vi "Main - bkp.vi"() -> ()   [LabVIEW 2013]
uses:
  <vilib>/Utility/error.llb/DialogType.ctl
  <vilib>/Utility/miscctls.llb/LVFontTypeDef.ctl
panel:
  out "Buv con ID":refnum<k5>
  out "LoadVolt":bool
  out "LoadPhase":bool
  in  "Tab Control":enum32{"ЛИНЗЫ ПОСТ. ТОКА", "ЛИНЗЫ ИМПУЛЬСНЫЕ"}(tab)
  in  "List of channels":i32(listbox)
  in  "ReadFromFile":bool
  in  "WriteToFile":bool
  out "Дата":string
  out "Время":string
  in  "Comm. current %":dbl=0.5 caption="А" min=0.0 max=72.0 step=0.25
  in  "Common curr. dec":bool
  in  "Common curr. inc":bool
  in  "ConnectAll":bool
  in  "DisconnectAll":bool
  in  "Set Output ON All":bool caption="ВЫХОДЫ ИСТОЧНИКОВ"
  out "текущий ист.":u8
  in  "SetCurrent":dbl min=0.0 max=72.0 step=0.1 format="%#.1g"
  in  "SetVoltage":dbl min=0.0 max=30.0 step=0.1 format="%#.1g"
  in  "SetCurrentB":bool
  in  "SetVoltageB":bool
  in  "SetOutputOffB":bool
  in  "SetOutputOnB":bool
  in  "ConnectChannel":bool
  in  "DisconnectChannel":bool
  in  "SetPhaseEn":bool=TRUE
  in  "BuvPhaseSetB":bool
  in  "SelectedBuvPhase":u16=7000 max=1000 step=1
  out "текущий ист. БУВ":u8
  in  "SelectedBuvOutVolt":dbl min=0.0 max=1000.0 step=0.1 format="%.1f"
  in  "SelectedBuvSetVolB":bool
  in  "Buv Table":i32(listbox)
  in  "Quit":bool=TRUE
  in  "SetCurrentAll":bool
  in  "SetVoltageAll":bool
  in  "Comm. voltage %":dbl caption="%" min=0.0 max=100.0 step=0.5
  in  "Common volt. dec":bool
  in  "Common volt. inc":bool
  in  "№":string="55"
  in  "DeleteChannel":bool
  in  "IP":string="172.16.21.19"
  in  "AddChannel":bool
  out "CURRENTSET":dbl[](array[numeric])
  in  "CurrentModulationOn":bool
  in  "Amp":dbl
  in  "CurrentModulationB":bool
  out "NAME":string[](array[string])
  out "ADRESS":string[](array[string])
  out "Measure_VI":refnum<vi>[](array[refnum])
  # "ВСЕ ИСТОЧНИКИ"
  # "ИСТОЧНИК №_"
  # "ИСТОЧНИК №_"
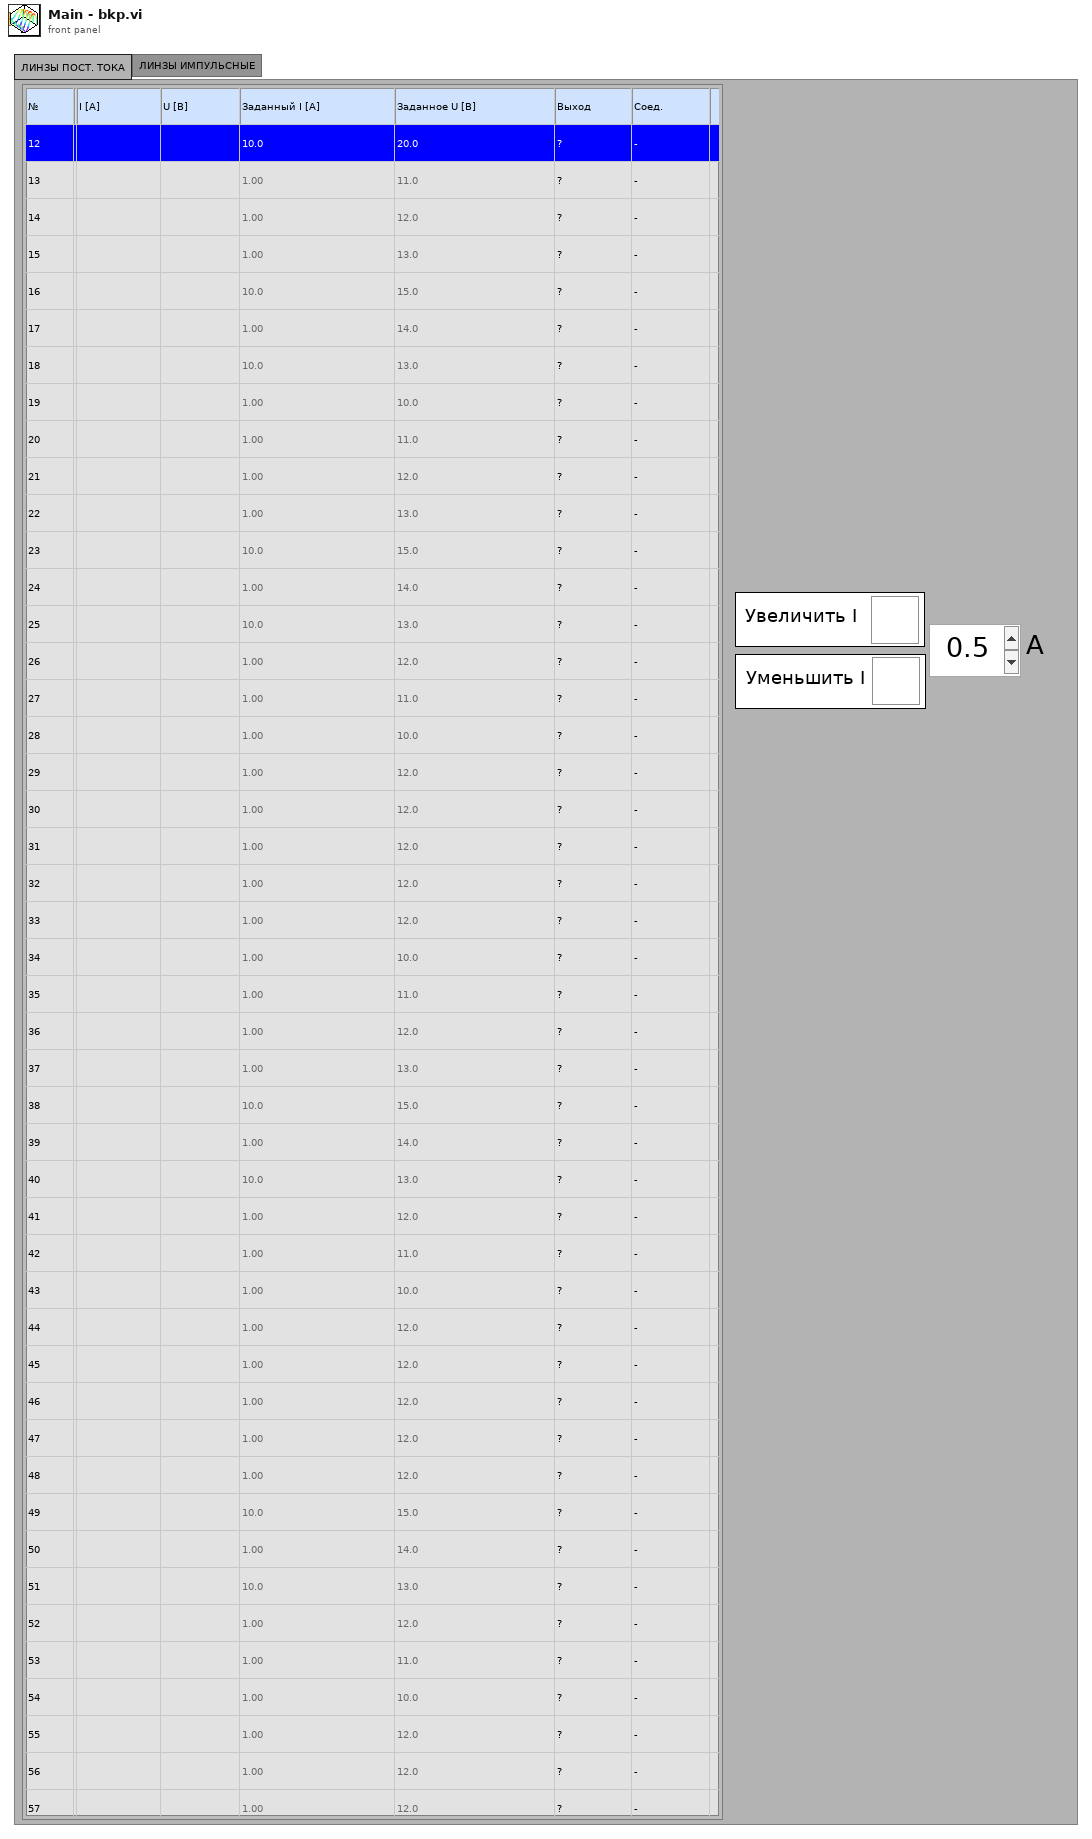
[diagram p1: front panel]
types:
  T1 = enum16{"open", "replace", "create", "open or create", "replace or create", "replace or create with confirmation"}
  T2 = enum8{"Enabled", "Disabled", "Disabled and Grayed Out"}
  T3 = typedef "DialogType.ctl" = u16
  T4 = typedef "LVFontTypeDef.ctl" = cluster{"Font Name":string, "Size":u16, "Bold":bool, "Italic":bool, "Underline":bool, "Strikeout":bool, "Color":u32}
  T5 = enum16{"Standard", "Buffered", "CRLF", "Immediate"}
  T6 = cluster{"milliseconds to wait":i32, "milliseconds to wait":i32}
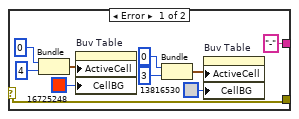
[diagram p6: hidden frame]
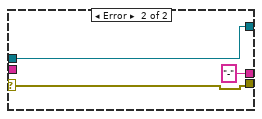
[diagram p7: hidden frame]
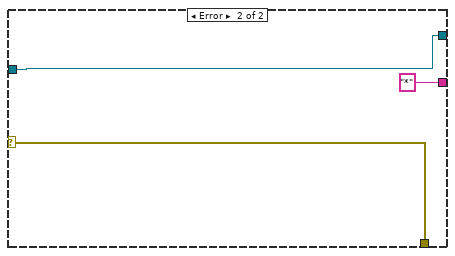
[diagram p8: hidden frame]
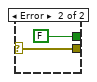
[diagram p10: hidden frame]
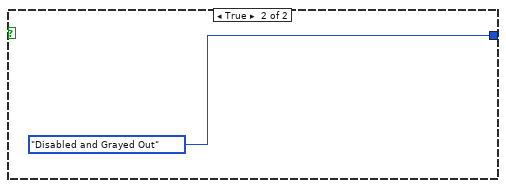
[diagram p11: hidden frame]
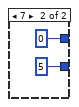
[diagram p13: hidden frame]
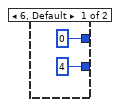
[diagram p14: hidden frame]
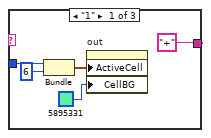
[diagram p15: hidden frame]
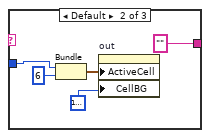
[diagram p16: hidden frame]
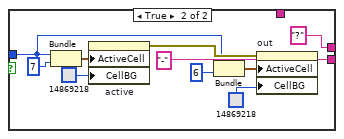
[diagram p17: hidden frame]
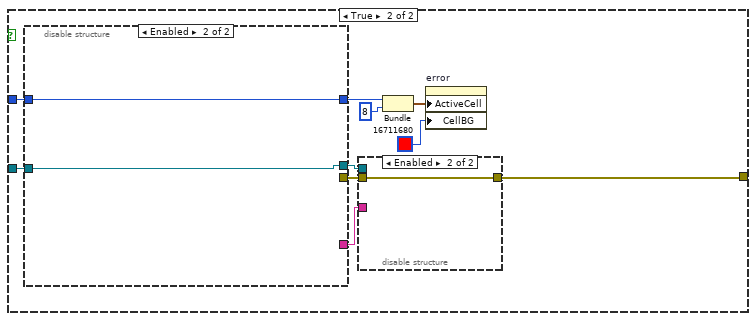
[diagram p18: hidden frame]
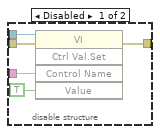
[diagram p19: hidden frame]
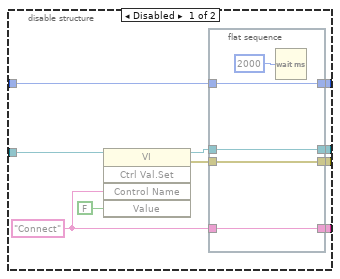
[diagram p20: hidden frame]
diagram:
  w38 = u8 0 ("Disabled")
  w40 = FALSE ("SetOutputOnB")
  w41 = FALSE ("OK Button")
  n1 = event shown="[0] \"Quit\": Value Change" {
    selector: _ -> [_]
    dyn-events: _ -> [_]
    timeout: _ -> [_]
    event "Quit": Value Change {
      n2 = event-data() -> ()  [unwired: 1 in, 1 out]
      n3 = flat-sequence {
        frame #0 {
          w46 = T3 0 items=["no dialog", "OK message", "continue or stop message", "OK message + warnings", "continue/stop + warnings"] ("type of dialog (OK msg:1)")
          n4 = local read "Measure_VI"() -> (w52:refnum<vi>[])
          n5 = local read "Buv con ID"() -> (w50:refnum<k5>)
          n6 = Array Size(array=w52) -> (size(s)=w51:i32)
          n7 = for {
            N: w51 -> [_]
            tunnel: [w53] -> w49 mode=indexing
            i -> [w54]
            n8 = local read "Measure_VI"() -> (w57:refnum<vi>[])
            n9 = Index Array(array=w57, index=w54) -> (element=w56:refnum<vi>)
            n10 = invoke class="VI" method="Ctrl Val.Set"(reference=w56, "Control Name"="Connect", "Value"=FALSE ("OK Button")) -> (error out=w53:errorcluster)  [unwired: 2 in, 4 out]
          }
          n11 = TCP Close Connection(connection ID=w50) -> (error out=w48:errorcluster)  [unwired: 2 in, 1 out]
          n12 = Merge Errors(w49, w48) -> (w47:errorcluster)
          n13 = call <vilib>:"General Error Handler.vi"("type of dialog (OK msg:1)"=w46, "error in (no error)"=w47) -> ()  [unwired: 9 in, 5 out]
        }
        frame #1 {
        }
        frame #2 {
          n14 = Stop(stop? (T)=TRUE) -> ()
        }
      }
    }
  }
  n15 = while {
    stop <- FALSE stop-if-true
    n16 = property on="List of channels" class="MCListbox (strict)"() -> ("ItemNames"=w66:string[][])  [unwired: 2 in, 2 out]
    n17 = Get Date/Time String(want seconds? (F)=TRUE) -> (date string=→"Дата":string, time string=→"Время":string)  [unwired: 2 in]
    n18 = Wait Until Next ms Multiple(millisecond multiple=u16 1000) -> ()  [unwired: 1 out]
    n19 = Empty Array?(array=w66) -> (empty?=w65:bool)
    n20 = case shown="False" w65 {
      tunnel: [T2."Enabled" ("Disabled") T2."Disabled and Grayed Out" ("Disabled")] -> w60
      frame False {
      }
      frame True {
      }
    }
    n21 = property on="Common curr. inc" class="Bool (strict)"("DisabledEnum"=w60) -> ()  [unwired: 2 in, 2 out]
    n22 = property on="Common curr. dec" class="Bool (strict)"("DisabledEnum"=w60) -> ()  [unwired: 2 in, 2 out]
    n23 = property on="Set Output ON All" class="Bool (strict)"("DisabledEnum"=w60) -> ()  [unwired: 2 in, 2 out]
    n24 = property on="Common volt. inc" class="Bool (strict)"("DisabledEnum"=w60) -> ()  [unwired: 2 in, 2 out]
    n25 = property on="DisconnectAll" class="Bool (strict)"("DisabledEnum"=w60) -> ()  [unwired: 2 in, 2 out]
    n26 = property on="SetVoltageB" class="Bool (strict)"("DisabledEnum"=w60) -> ()  [unwired: 2 in, 2 out]
    n27 = property on="ConnectChannel" class="Bool (strict)"("DisabledEnum"=w60) -> ()  [unwired: 2 in, 2 out]
    n28 = property on="SetOutputOnB" class="Bool (strict)"("DisabledEnum"=w60) -> ()  [unwired: 2 in, 2 out]
    n29 = property on="DisconnectChannel" class="Bool (strict)"("DisabledEnum"=w60) -> ()  [unwired: 2 in, 2 out]
    n30 = property on="SetOutputOffB" class="Bool (strict)"("DisabledEnum"=w60) -> ()  [unwired: 2 in, 2 out]
    n31 = property on="ConnectAll" class="Bool (strict)"("DisabledEnum"=w60) -> ()  [unwired: 2 in, 2 out]
    n32 = property on="SetCurrentB" class="Bool (strict)"("DisabledEnum"=w60) -> ()  [unwired: 2 in, 2 out]
  }
  n33 = while {
    stop <- FALSE stop-if-true
    n34 = event shown="[16] \"WriteToFile\": Value Change" {
      selector: _ -> [_ _ _ _ _ _ _ _ _ _ _ _ _ _ _ _ _ _ _ _]
      dyn-events: _ -> [_ _ _ _ _ _ _ _ _ _ _ _ _ _ _ _ _ _ _ _]
      timeout: _ -> [_ _ _ _ _ _ _ _ _ _ _ _ _ _ _ _ _ _ _ _]
      tunnel: [w73 _ _ _ w177 w193 w209 w250 w291 w306 w332 w348 w364 w381 w402 w425 w443 w494 w571 w594] -> w70
      event "AddChannel": Value Change {
        n35 = event-data() -> ()  [unwired: 7 out]
        n36 = flat-sequence {
          tunnel: [w76] -> w74
          tunnel: [w86] -> w73
          tunnel: w74 -> [w86]
          frame #0 {
            w75 = u8 2 ("Disabled")
            n37 = property on="Quit" class="Bool (strict)"("Disabled"=w75) -> ()  [unwired: 2 in, 2 out]
            n38 = property on="AddChannel" class="Bool (strict)"("Disabled"=w75) -> ()  [unwired: 2 in, 2 out]
            n39 = property on="CurrentModulationB" class="Bool (strict)"("Disabled"=w75) -> ()  [unwired: 2 in, 2 out]
            n40 = property on="DisconnectChannel" class="Bool (strict)"("Disabled"=w75) -> ()  [unwired: 2 in, 2 out]
            n41 = property on="ConnectAll" class="Bool (strict)"("Disabled"=w75) -> ()  [unwired: 2 in, 2 out]
            n42 = property on="ReadFromFile" class="Bool (strict)"("Disabled"=w75) -> ()  [unwired: 2 in, 2 out]
            n43 = property on="ConnectChannel" class="Bool (strict)"("Disabled"=w75) -> ()  [unwired: 2 in, 2 out]
            n44 = property on="DeleteChannel" class="Bool (strict)"("Disabled"=w75) -> ()  [unwired: 2 in, 2 out]
            n45 = property on="SetOutputOnB" class="Bool (strict)"("Disabled"=w75) -> ()  [unwired: 2 in, 2 out]
            n46 = property on="Set Output ON All" class="Bool (strict)"("Disabled"=w75) -> ()  [unwired: 2 in, 2 out]
            n47 = property on="SetVoltageB" class="Bool (strict)"("Disabled"=w75) -> ()  [unwired: 2 in, 2 out]
            n48 = property on="SetOutputOffB" class="Bool (strict)"("Disabled"=w75) -> ()  [unwired: 2 in, 2 out]
            n49 = property on="SetVoltageAll" class="Bool (strict)"("Disabled"=w75) -> ()  [unwired: 2 in, 2 out]
            n50 = property on="SetCurrentAll" class="Bool (strict)"("Disabled"=w75) -> ()  [unwired: 2 in, 2 out]
            n51 = property on="DisconnectAll" class="Bool (strict)"("Disabled"=w75) -> ()  [unwired: 2 in, 2 out]
            n52 = property on="WriteToFile" class="Bool (strict)"("Disabled"=w75) -> ()  [unwired: 2 in, 2 out]
            n53 = property on="SetCurrentB" class="Bool (strict)"("Disabled"=w75) -> ()  [unwired: 2 in, 2 out]
          }
          frame #1 {
            w77 = 0.0 ("SetVoltage")
            n54 = local read "Measure_VI"() -> (w81:refnum<vi>[])
            n55 = local read "ADRESS"() -> (w83:string[])
            n56 = local read "NAME"() -> (w82:string[])
            n57 = call "AddChannel.vi"("VIRef"=w81, "Name"="№", "SetCurrent"=w77, "ADRESS"=w83, "NAME"=w82, "Address"="IP", "SetVoltage"=w77) -> ("NAMEOut"=w78:string[], "error out"=w76:errorcluster, "ADRESSOut"=w79:string[], "VIRefOut"=w80:refnum<vi>[])  [unwired: 1 in, 4 out]
            n58 = local write "NAME"(w78) -> ()
            n59 = local write "ADRESS"(w79) -> ()
            n60 = local write "Measure_VI"(w80) -> ()
          }
          frame #2 {
            w87 = u8 0 ("Disabled")
            n61 = local write "AddChannel"(FALSE ("AddChannel")) -> ()
            n62 = property on="Quit" class="Bool (strict)"("Disabled"=w87) -> ()  [unwired: 2 in, 2 out]
            n63 = property on="AddChannel" class="Bool (strict)"("Disabled"=w87) -> ()  [unwired: 2 in, 2 out]
            n64 = property on="CurrentModulationB" class="Bool (strict)"("Disabled"=w87) -> ()  [unwired: 2 in, 2 out]
            n65 = property on="DisconnectChannel" class="Bool (strict)"("Disabled"=w87) -> ()  [unwired: 2 in, 2 out]
            n66 = property on="ReadFromFile" class="Bool (strict)"("Disabled"=w87) -> ()  [unwired: 2 in, 2 out]
            n67 = property on="ConnectChannel" class="Bool (strict)"("Disabled"=w87) -> ()  [unwired: 2 in, 2 out]
            n68 = property on="DeleteChannel" class="Bool (strict)"("Disabled"=w87) -> ()  [unwired: 2 in, 2 out]
            n69 = property on="SetVoltageB" class="Bool (strict)"("Disabled"=w87) -> ()  [unwired: 2 in, 2 out]
            n70 = property on="Set Output ON All" class="Bool (strict)"("Disabled"=w87) -> ()  [unwired: 2 in, 2 out]
            n71 = property on="SetOutputOffB" class="Bool (strict)"("Disabled"=w87) -> ()  [unwired: 2 in, 2 out]
            n72 = property on="ConnectAll" class="Bool (strict)"("Disabled"=w87) -> ()  [unwired: 2 in, 2 out]
            n73 = property on="SetVoltageAll" class="Bool (strict)"("Disabled"=w87) -> ()  [unwired: 2 in, 2 out]
            n74 = property on="SetCurrentAll" class="Bool (strict)"("Disabled"=w87) -> ()  [unwired: 2 in, 2 out]
            n75 = property on="DisconnectAll" class="Bool (strict)"("Disabled"=w87) -> ()  [unwired: 2 in, 2 out]
            n76 = property on="WriteToFile" class="Bool (strict)"("Disabled"=w87) -> ()  [unwired: 2 in, 2 out]
            n77 = property on="SetCurrentB" class="Bool (strict)"("Disabled"=w87) -> ()  [unwired: 2 in, 2 out]
            n78 = property on="SetOutputOnB" class="Bool (strict)"("Disabled"=w87) -> ()  [unwired: 2 in, 2 out]
          }
        }
      }
      event "List of channels": Mouse Down {
        # "Работа с выбранным источником"
        n79 = event-data() -> ()  [unwired: 2 out]
        n80 = property on="List of channels" class="MCListbox (strict)"() -> ("ItemNames"=w92:string[][])  [unwired: 2 in, 2 out]
        n81 = property on="List of channels" class="MCListbox (strict)"() -> ("Value"=w91:i32)  [unwired: 2 in, 2 out]
        n82 = Index Array(array=w92, index (row)=w91) -> (element=w90:string[])  [unwired: 1 in]
        n83 = Empty Array?(array=w90) -> (empty?=w89:bool)
        n84 = case shown="False" w89 {
          tunnel: w90 -> [w93 _]
          frame False {
            n85 = flat-sequence {
              tunnel: w93 -> [w99]
              tunnel: [w99] -> w94
              tunnel: w94 -> [w112]
              frame #0 {
                n86 = Index Array(array=w99, index=0) -> (element=w102:string)
                n87 = Index Array(array=w99, index=7) -> (element=w100:string)
                n88 = case shown="\"-\", Default" w100 {
                  tunnel: [T2."Enabled" ("Disabled") T2."Disabled and Grayed Out" ("Disabled")] -> w95
                  tunnel: [w106 w108] -> w96
                  tunnel: [w106 w108] -> w98
                  tunnel: [w106 w108] -> w97
                  frame "-", Default {
                    w106 = T2."Disabled and Grayed Out" ("Disabled")
                  }
                  frame "+" {
                    w108 = T2."Enabled" ("Disabled")
                    # "соединение с ист."
                  }
                }
                n89 = Scan From String(format string="%f", input string=w102) -> (output 1=→"текущий ист.":u8)  [unwired: 3 in, 3 out]
                n90 = property on="DisconnectAll" class="Bool (strict)"("DisabledEnum"=w96) -> ()  [unwired: 2 in, 2 out]
                n91 = property on="DisconnectChannel" class="Bool (strict)"("DisabledEnum"=w96) -> ()  [unwired: 2 in, 2 out]
                n92 = property on="SetOutputOffB" class="Bool (strict)"("DisabledEnum"=w98) -> ()  [unwired: 2 in, 2 out]
                n93 = property on="SetOutputOnB" class="Bool (strict)"("DisabledEnum"=w97) -> ()  [unwired: 2 in, 2 out]
                n94 = property on="ConnectChannel" class="Bool (strict)"("DisabledEnum"=w95) -> ()  [unwired: 2 in, 2 out]
                n95 = property on="ConnectAll" class="Bool (strict)"("DisabledEnum"=w95) -> ()  [unwired: 2 in, 2 out]
              }
              frame #1 {
                n96 = Index Array(array=w112, index=5) -> (element=w117:string)
                n97 = Index Array(array=w112, index=6) -> (element=w120:string)
                n98 = Index Array(array=w112, index=4) -> (element=w114:string)
                n99 = case shown="\"-\", Default" w120 {
                  tunnel: [T2."Enabled" ("Disabled") T2."Disabled and Grayed Out" ("Disabled") w127] -> w121
                  tunnel: [T2."Disabled and Grayed Out" ("Disabled") T2."Enabled" ("Disabled") w127] -> w122
                  frame "-", Default {
                  }
                  frame "+" {
                  }
                  frame "?" {
                    w127 = T2."Disabled and Grayed Out" ("Disabled")
                  }
                }
                n100 = Scan From String(format string="%f", input string=w117) -> (output 1=w110:dbl)  [unwired: 3 in, 3 out]
                n101 = Scan From String(format string="%f", input string=w114) -> (output 1=w111:dbl)  [unwired: 3 in, 3 out]
                n102 = local write "SetVoltage"(w110) -> ()
                n103 = local write "SetCurrent"(w111) -> ()
                n104 = property on="SetOutputOffB" class="Bool (strict)"("DisabledEnum"=w122) -> ()  [unwired: 2 in, 2 out]
                n105 = property on="SetOutputOnB" class="Bool (strict)"("DisabledEnum"=w121) -> ()  [unwired: 2 in, 2 out]
              }
            }
          }
          frame True {
          }
        }
      }
      event "Buv Table": Mouse Down {
        # "Работа с выбранным источником БУВ"
        n106 = event-data() -> ()  [unwired: 2 out]
        n107 = property on="Buv Table" class="MCListbox (strict)"() -> ("ItemNames"=w131:string[][])  [unwired: 2 in, 2 out]
        n108 = property on="Buv Table" class="MCListbox (strict)"() -> ("Value"=w130:i32)  [unwired: 2 in, 2 out]
        n109 = Index Array(array=w131, index (row)=w130) -> (element=w129:string[])  [unwired: 1 in]
        n110 = Empty Array?(array=w129) -> (empty?=w128:bool)
        n111 = case shown="False" w128 {
          tunnel: w129 -> [w132 _]
          frame False {
            n112 = flat-sequence {
              tunnel: w132 -> [w135]
              tunnel: [w135] -> w133
              tunnel: w133 -> [w145]
              frame #0 {
                n113 = Index Array(array=w135, index=3) -> (element=w136:string)
                n114 = Index Array(array=w135, index=0) -> (element=w138:string)
                n115 = case shown="\"+\"" w136 {
                  frame "-", Default {
                  }
                  frame "+" {
                    # "соединение с ист."
                  }
                }
                n116 = Scan From String(format string="%f", input string=w138) -> (output 1=→"текущий ист. БУВ":u8)  [unwired: 3 in, 3 out]
              }
              frame #1 {
                n117 = disable-structure shown="Disabled" {
                  disable-tunnel: w145 -> [w147 _]
                  frame Disabled {
                    n118 = Index Array(array=w147, index=1) -> (element=w148:string)
                    n119 = Scan From String(format string="%f", input string=w148) -> ()  [unwired: 4 in, 3 out]
                  }
                  frame Enabled {
                  }
                }
                n120 = Index Array(array=w145, index=2) -> (element=w143:string)
                n121 = Scan From String(format string="%f", input string=w143) -> (output 1=w141:dbl)  [unwired: 3 in, 3 out]
                n122 = local write "SelectedBuvOutVolt"(w141) -> ()
              }
            }
          }
          frame True {
          }
        }
      }
      event Panel Close? {
        n123 = event-data() -> ()  [unwired: 5 out]
        n124 = Two Button Dialog(message="Вы уверены, что хотите закрыть программу?", 1:"Нет" ("F button name (\"Cancel\")"), 2:"Да" ("T button name (\"OK\")")) -> (T button?=w153:bool)
        n125 = case shown="True" w153 {
          frame False {
          }
          frame True {
            n126 = disable-structure shown="Disabled" {
              frame Disabled {
                n127 = local read item#-1() -> (w163)
                n128 = TCP Close Connection(connection ID=w163) -> ()  [unwired: 2 in, 2 out]
              }
              frame Enabled {
              }
            }
            n129 = local read "Measure_VI"() -> (w155:refnum<vi>[])
            n130 = Array Size(array=w155) -> (size(s)=w154:i32)
            n131 = for {
              N: w154 -> [_]
              tunnel: w155 -> [w173]
              tunnel: [w171] -> w162 mode=indexing
              i -> [w174]
              n132 = Index Array(array=w173, index=w174) -> (element=w172:refnum<vi>)
              n133 = invoke class="VI" method="Ctrl Val.Set"(reference=w172, "Control Name"="Connect", "Value"=FALSE) -> (error out=w171:errorcluster)  [unwired: 2 in, 4 out]
            }
            n134 = flat-sequence {
              tunnel: [w165] -> w161
              tunnel: w162 -> [w165]
              frame #0 {
                n135 = Wait (ms)(milliseconds to wait=u32 1000) -> ()  [unwired: 1 out]
              }
            }
            n136 = local read "Measure_VI"() -> (w156:refnum<vi>[])
            n137 = Array Size(array=w156) -> (size(s)=w157:i32)
            n138 = for {
              N: w157 -> [_]
              tunnel: w156 -> [w169]
              tunnel: [w167] -> w158 mode=indexing
              tunnel: w161 -> [w166] mode=indexing
              i -> [w170]
              n139 = Index Array(array=w169, index=w170) -> (element=w168:refnum<vi>)
              n140 = invoke class="VI" method="Abort VI"(reference=w168, error in=w166) -> (error out=w167:errorcluster)  [unwired: 1 in, 2 out]
            }
            n141 = Merge Errors(w158) -> (w159:errorcluster)
            n142 = call <vilib>:"General Error Handler.vi"("type of dialog (OK msg:1)"=u32 0 ("milliseconds to wait"), "error in (no error)"=w159) -> ()  [unwired: 9 in, 5 out]
          }
        }
        n143 = event-data() -> ()  [unwired: 2 in, 1 out]
      }
      event "SetVoltageAll": Value Change {
        n144 = event-data() -> ()  [unwired: 7 out]
        n145 = flat-sequence {
          tunnel: [w181] -> w179
          tunnel: [w190] -> w178
          tunnel: w179 -> [w190]
          frame #0 {
            w180 = u8 2 ("Disabled")
            n146 = property on="Quit" class="Bool (strict)"("Disabled"=w180) -> ()  [unwired: 2 in, 2 out]
            n147 = property on="AddChannel" class="Bool (strict)"("Disabled"=w180) -> ()  [unwired: 2 in, 2 out]
            n148 = property on="CurrentModulationB" class="Bool (strict)"("Disabled"=w180) -> ()  [unwired: 2 in, 2 out]
            n149 = property on="DisconnectChannel" class="Bool (strict)"("Disabled"=w180) -> ()  [unwired: 2 in, 2 out]
            n150 = property on="ConnectAll" class="Bool (strict)"("Disabled"=w180) -> ()  [unwired: 2 in, 2 out]
            n151 = property on="ReadFromFile" class="Bool (strict)"("Disabled"=w180) -> ()  [unwired: 2 in, 2 out]
            n152 = property on="ConnectChannel" class="Bool (strict)"("Disabled"=w180) -> ()  [unwired: 2 in, 2 out]
            n153 = property on="DeleteChannel" class="Bool (strict)"("Disabled"=w180) -> ()  [unwired: 2 in, 2 out]
            n154 = property on="SetVoltageB" class="Bool (strict)"("Disabled"=w180) -> ()  [unwired: 2 in, 2 out]
            n155 = property on="Set Output ON All" class="Bool (strict)"("Disabled"=w180) -> ()  [unwired: 2 in, 2 out]
            n156 = property on="SetOutputOffB" class="Bool (strict)"("Disabled"=w180) -> ()  [unwired: 2 in, 2 out]
            n157 = property on="SetVoltageAll" class="Bool (strict)"("Disabled"=w180) -> ()  [unwired: 2 in, 2 out]
            n158 = property on="SetCurrentAll" class="Bool (strict)"("Disabled"=w180) -> ()  [unwired: 2 in, 2 out]
            n159 = property on="DisconnectAll" class="Bool (strict)"("Disabled"=w180) -> ()  [unwired: 2 in, 2 out]
            n160 = property on="WriteToFile" class="Bool (strict)"("Disabled"=w180) -> ()  [unwired: 2 in, 2 out]
            n161 = property on="SetCurrentB" class="Bool (strict)"("Disabled"=w180) -> ()  [unwired: 2 in, 2 out]
            n162 = property on="SetOutputOnB" class="Bool (strict)"("Disabled"=w180) -> ()  [unwired: 2 in, 2 out]
          }
          frame #1 {
            n163 = local read "Measure_VI"() -> (w183:refnum<vi>[])
            n164 = Array Size(array=w183) -> (size(s)=w182:i32)
            n165 = for {
              N: w182 -> [_]
              tunnel: [w184] -> w181 mode=indexing
              i -> [w186]
              n166 = local read "Measure_VI"() -> (w189:refnum<vi>[])
              n167 = Index Array(array=w189, index=w186) -> (element=w185:refnum<vi>)
              n168 = invoke class="VI" method="Ctrl Val.Set"(reference=w185, "Control Name"="NeedToSetVoltage", "Value"=TRUE ("ConnectChannel")) -> (error out=w184:errorcluster)  [unwired: 2 in, 4 out]
            }
          }
          frame #2 {
            w191 = u8 0 ("Disabled")
            n169 = local write "SetVoltageAll"(FALSE ("SetVoltageAll")) -> ()
            n170 = property on="Quit" class="Bool (strict)"("Disabled"=w191) -> ()  [unwired: 2 in, 2 out]
            n171 = property on="AddChannel" class="Bool (strict)"("Disabled"=w191) -> ()  [unwired: 2 in, 2 out]
            n172 = property on="CurrentModulationB" class="Bool (strict)"("Disabled"=w191) -> ()  [unwired: 2 in, 2 out]
            n173 = property on="DisconnectChannel" class="Bool (strict)"("Disabled"=w191) -> ()  [unwired: 2 in, 2 out]
            n174 = property on="ReadFromFile" class="Bool (strict)"("Disabled"=w191) -> ()  [unwired: 2 in, 2 out]
            n175 = property on="ConnectChannel" class="Bool (strict)"("Disabled"=w191) -> ()  [unwired: 2 in, 2 out]
            n176 = property on="DeleteChannel" class="Bool (strict)"("Disabled"=w191) -> ()  [unwired: 2 in, 2 out]
            n177 = property on="WriteToFile" class="Bool (strict)"("Disabled"=w191) -> ()  [unwired: 2 in, 2 out]
            n178 = property on="Set Output ON All" class="Bool (strict)"("Disabled"=w191) -> ()  [unwired: 2 in, 2 out]
            n179 = property on="SetCurrentB" class="Bool (strict)"("Disabled"=w191) -> ()  [unwired: 2 in, 2 out]
            n180 = property on="ConnectAll" class="Bool (strict)"("Disabled"=w191) -> ()  [unwired: 2 in, 2 out]
            n181 = property on="SetOutputOnB" class="Bool (strict)"("Disabled"=w191) -> ()  [unwired: 2 in, 2 out]
            n182 = property on="SetVoltageB" class="Bool (strict)"("Disabled"=w191) -> ()  [unwired: 2 in, 2 out]
            n183 = property on="SetOutputOffB" class="Bool (strict)"("Disabled"=w191) -> ()  [unwired: 2 in, 2 out]
            n184 = property on="SetVoltageAll" class="Bool (strict)"("Disabled"=w191) -> ()  [unwired: 2 in, 2 out]
            n185 = property on="SetCurrentAll" class="Bool (strict)"("Disabled"=w191) -> ()  [unwired: 2 in, 2 out]
            n186 = property on="DisconnectAll" class="Bool (strict)"("Disabled"=w191) -> ()  [unwired: 2 in, 2 out]
          }
        }
        n187 = Merge Errors(w178) -> (w177:errorcluster)
      }
      event "SetCurrentAll": Value Change {
        n188 = event-data() -> ()  [unwired: 7 out]
        n189 = flat-sequence {
          tunnel: [w197] -> w195
          tunnel: [w206] -> w194
          tunnel: w195 -> [w206]
          frame #0 {
            w196 = u8 2 ("Disabled")
            n190 = property on="Quit" class="Bool (strict)"("Disabled"=w196) -> ()  [unwired: 2 in, 2 out]
            n191 = property on="AddChannel" class="Bool (strict)"("Disabled"=w196) -> ()  [unwired: 2 in, 2 out]
            n192 = property on="CurrentModulationB" class="Bool (strict)"("Disabled"=w196) -> ()  [unwired: 2 in, 2 out]
            n193 = property on="DisconnectChannel" class="Bool (strict)"("Disabled"=w196) -> ()  [unwired: 2 in, 2 out]
            n194 = property on="ConnectAll" class="Bool (strict)"("Disabled"=w196) -> ()  [unwired: 2 in, 2 out]
            n195 = property on="ReadFromFile" class="Bool (strict)"("Disabled"=w196) -> ()  [unwired: 2 in, 2 out]
            n196 = property on="ConnectChannel" class="Bool (strict)"("Disabled"=w196) -> ()  [unwired: 2 in, 2 out]
            n197 = property on="DeleteChannel" class="Bool (strict)"("Disabled"=w196) -> ()  [unwired: 2 in, 2 out]
            n198 = property on="SetOutputOffB" class="Bool (strict)"("Disabled"=w196) -> ()  [unwired: 2 in, 2 out]
            n199 = property on="Set Output ON All" class="Bool (strict)"("Disabled"=w196) -> ()  [unwired: 2 in, 2 out]
            n200 = property on="SetVoltageAll" class="Bool (strict)"("Disabled"=w196) -> ()  [unwired: 2 in, 2 out]
            n201 = property on="SetCurrentAll" class="Bool (strict)"("Disabled"=w196) -> ()  [unwired: 2 in, 2 out]
            n202 = property on="DisconnectAll" class="Bool (strict)"("Disabled"=w196) -> ()  [unwired: 2 in, 2 out]
            n203 = property on="WriteToFile" class="Bool (strict)"("Disabled"=w196) -> ()  [unwired: 2 in, 2 out]
            n204 = property on="SetCurrentB" class="Bool (strict)"("Disabled"=w196) -> ()  [unwired: 2 in, 2 out]
            n205 = property on="SetOutputOnB" class="Bool (strict)"("Disabled"=w196) -> ()  [unwired: 2 in, 2 out]
            n206 = property on="SetVoltageB" class="Bool (strict)"("Disabled"=w196) -> ()  [unwired: 2 in, 2 out]
          }
          frame #1 {
            n207 = local read "Measure_VI"() -> (w199:refnum<vi>[])
            n208 = Array Size(array=w199) -> (size(s)=w198:i32)
            n209 = for {
              N: w198 -> [_]
              tunnel: [w200] -> w197 mode=indexing
              i -> [w202]
              n210 = local read "Measure_VI"() -> (w205:refnum<vi>[])
              n211 = Index Array(array=w205, index=w202) -> (element=w201:refnum<vi>)
              n212 = invoke class="VI" method="Ctrl Val.Set"(reference=w201, "Control Name"="NeedToSetCurrent", "Value"=TRUE ("ConnectChannel")) -> (error out=w200:errorcluster)  [unwired: 2 in, 4 out]
            }
          }
          frame #2 {
            w207 = u8 0 ("Disabled")
            n213 = local write "SetCurrentAll"(FALSE ("SetVoltageAll")) -> ()
            n214 = property on="Quit" class="Bool (strict)"("Disabled"=w207) -> ()  [unwired: 2 in, 2 out]
            n215 = property on="AddChannel" class="Bool (strict)"("Disabled"=w207) -> ()  [unwired: 2 in, 2 out]
            n216 = property on="CurrentModulationB" class="Bool (strict)"("Disabled"=w207) -> ()  [unwired: 2 in, 2 out]
            n217 = property on="DisconnectChannel" class="Bool (strict)"("Disabled"=w207) -> ()  [unwired: 2 in, 2 out]
            n218 = property on="ReadFromFile" class="Bool (strict)"("Disabled"=w207) -> ()  [unwired: 2 in, 2 out]
            n219 = property on="ConnectChannel" class="Bool (strict)"("Disabled"=w207) -> ()  [unwired: 2 in, 2 out]
            n220 = property on="DeleteChannel" class="Bool (strict)"("Disabled"=w207) -> ()  [unwired: 2 in, 2 out]
            n221 = property on="WriteToFile" class="Bool (strict)"("Disabled"=w207) -> ()  [unwired: 2 in, 2 out]
            n222 = property on="Set Output ON All" class="Bool (strict)"("Disabled"=w207) -> ()  [unwired: 2 in, 2 out]
            n223 = property on="SetCurrentB" class="Bool (strict)"("Disabled"=w207) -> ()  [unwired: 2 in, 2 out]
            n224 = property on="ConnectAll" class="Bool (strict)"("Disabled"=w207) -> ()  [unwired: 2 in, 2 out]
            n225 = property on="SetOutputOnB" class="Bool (strict)"("Disabled"=w207) -> ()  [unwired: 2 in, 2 out]
            n226 = property on="SetVoltageB" class="Bool (strict)"("Disabled"=w207) -> ()  [unwired: 2 in, 2 out]
            n227 = property on="SetOutputOffB" class="Bool (strict)"("Disabled"=w207) -> ()  [unwired: 2 in, 2 out]
            n228 = property on="SetVoltageAll" class="Bool (strict)"("Disabled"=w207) -> ()  [unwired: 2 in, 2 out]
            n229 = property on="SetCurrentAll" class="Bool (strict)"("Disabled"=w207) -> ()  [unwired: 2 in, 2 out]
            n230 = property on="DisconnectAll" class="Bool (strict)"("Disabled"=w207) -> ()  [unwired: 2 in, 2 out]
          }
        }
        n231 = Merge Errors(w194) -> (w193:errorcluster)
      }
      event "Common curr. inc", "Common curr. dec": Value Change {
        # "Увелич/уменьшение тока на всех ист"
        n232 = event-data() -> ()  [unwired: 2 out]
        n233 = local read "ADRESS"() -> (w212:string[])
        n234 = Array Size(array=w212) -> (size(s)=w213:i32)
        n235 = for {
          N: w213 -> [_]
          tunnel: [w223] -> w211 mode=indexing
          i -> [w237]
          n236 = local read "Measure_VI"() -> (w240:refnum<vi>[])
          n237 = Index Array(array=w240, index=w237) -> (element=w231:refnum<vi>)
          n238 = invoke class="VI" method="Ctrl Val.Get"(reference=w231, "Control Name"="SetCurrentStr") -> (reference out=w225:refnum<vi>, error out=w235:errorcluster, "Get Control Value Variant"=w239:variant)  [unwired: 2 in, 1 out]
          n239 = Variant To Data(error in=w235, type="" ("Control Name"), Variant=w239) -> (data=w234:string, error out=w233:errorcluster)
          n240 = Scan From String(format string="%f", input string=w234, error in=w233) -> (error out=w224:errorcluster, output 1=w222:dbl)  [unwired: 2 in, 2 out]
          n241 = local read "Common curr. inc"() -> (w221:bool)
          n242 = local read "Common curr. dec"() -> (w219:bool)
          n243 = case shown="True" w221 {
            tunnel: "Comm. current %" -> [w245 w249]
            tunnel: w222 -> [w246 w248]
            tunnel: [w246 w247] -> w220
            tunnel: [w245 _] -> w218
            frame False {
            }
            frame True {
              n244 = Add(x=w248, y=w249) -> (x+y=w247:dbl)
            }
          }
          n245 = case shown="True" w219 {
            tunnel: w220 -> [w241 w244]
            tunnel: [w241 w243] -> w217
            tunnel: w218 -> [_ w242]
            frame False {
            }
            frame True {
              n246 = Subtract(x=w244, y=w242) -> (x-y=w243:dbl)
            }
          }
          n247 = invoke class="VI" method="Ctrl Val.Set"(reference=w225, error in=w224, "Control Name"="SetCurrent", "Value"=w217) -> (reference out=w227:refnum<vi>, error out=w226:errorcluster)  [unwired: 1 in, 3 out]
          n248 = invoke class="VI" method="Ctrl Val.Set"(reference=w227, error in=w226, "Control Name"="NeedToSetCurrent", "Value"=TRUE ("ConnectChannel")) -> (error out=w223:errorcluster)  [unwired: 1 in, 4 out]
        }
        n249 = Merge Errors(w211) -> (w210:errorcluster)
        n250 = flat-sequence {
          tunnel: w210 -> [w215]
          tunnel: [w215] -> w209
          frame #0 {
            w214 = FALSE ("ConnectChannel")
            n251 = local write "Common curr. inc"(w214) -> ()
            n252 = local write "Common curr. dec"(w214) -> ()
          }
        }
      }
      event "Common volt. inc", "Common volt. dec": Value Change {
        # "Увелич/уменьшение тока на всех ист"
        n253 = event-data() -> ()  [unwired: 2 out]
        n254 = local read "ADRESS"() -> (w253:string[])
        n255 = Array Size(array=w253) -> (size(s)=w254:i32)
        n256 = for {
          N: w254 -> [_]
          tunnel: [w264] -> w252 mode=indexing
          i -> [w278]
          n257 = local read "Measure_VI"() -> (w281:refnum<vi>[])
          n258 = Index Array(array=w281, index=w278) -> (element=w272:refnum<vi>)
          n259 = invoke class="VI" method="Ctrl Val.Get"(reference=w272, "Control Name"="SetVoltageStr") -> (reference out=w266:refnum<vi>, error out=w276:errorcluster, "Get Control Value Variant"=w280:variant)  [unwired: 2 in, 1 out]
          n260 = Variant To Data(error in=w276, type="" ("Control Name"), Variant=w280) -> (data=w275:string, error out=w274:errorcluster)
          n261 = Scan From String(format string="%f", input string=w275, error in=w274) -> (error out=w265:errorcluster, output 1=w263:dbl)  [unwired: 2 in, 2 out]
          n262 = local read "Common volt. inc"() -> (w262:bool)
          n263 = local read "Common volt. dec"() -> (w260:bool)
          n264 = case shown="True" w262 {
            tunnel: "Comm. voltage %" -> [w286 w290]
            tunnel: w263 -> [w287 w289]
            tunnel: [w287 w288] -> w261
            tunnel: [w286 _] -> w259
            frame False {
            }
            frame True {
              n265 = Add(x=w289, y=w290) -> (x+y=w288:dbl)
            }
          }
          n266 = case shown="False" w260 {
            tunnel: w261 -> [w282 w285]
            tunnel: [w282 w284] -> w258
            tunnel: w259 -> [_ w283]
            frame False {
            }
            frame True {
              n267 = Subtract(x=w285, y=w283) -> (x-y=w284:dbl)
            }
          }
          n268 = invoke class="VI" method="Ctrl Val.Set"(reference=w266, error in=w265, "Control Name"="SetVoltage", "Value"=w258) -> (reference out=w268:refnum<vi>, error out=w267:errorcluster)  [unwired: 1 in, 3 out]
          n269 = invoke class="VI" method="Ctrl Val.Set"(reference=w268, error in=w267, "Control Name"="NeedToSetVoltage", "Value"=TRUE ("ConnectChannel")) -> (error out=w264:errorcluster)  [unwired: 1 in, 4 out]
        }
        n270 = Merge Errors(w252) -> (w251:errorcluster)
        n271 = flat-sequence {
          tunnel: w251 -> [w256]
          tunnel: [w256] -> w250
          frame #0 {
            w255 = FALSE ("ConnectChannel")
            n272 = local write "Common volt. inc"(w255) -> ()
            n273 = local write "Common volt. dec"(w255) -> ()
          }
        }
      }
      event "DisconnectChannel": Value Change {
        n274 = event-data() -> ()  [unwired: 7 out]
        n275 = property on="List of channels" class="MCListbox (strict)"() -> ("Value"=w295:i32)  [unwired: 2 in, 2 out]
        n276 = flat-sequence {
          tunnel: w295 -> [w297]
          tunnel: [w297] -> w294
          tunnel: w294 -> [w299]
          tunnel: [w298] -> w292
          tunnel: [w304] -> w293
          tunnel: w292 -> [w304]
          frame #0 {
            w296 = u8 2 ("Disabled")
            n277 = property on="AddChannel" class="Bool (strict)"("Disabled"=w296) -> ()  [unwired: 2 in, 2 out]
            n278 = property on="Set Output ON All" class="Bool (strict)"("Disabled"=w296) -> ()  [unwired: 2 in, 2 out]
            n279 = property on="CurrentModulationB" class="Bool (strict)"("Disabled"=w296) -> ()  [unwired: 2 in, 2 out]
            n280 = property on="ConnectAll" class="Bool (strict)"("Disabled"=w296) -> ()  [unwired: 2 in, 2 out]
            n281 = property on="DisconnectChannel" class="Bool (strict)"("Disabled"=w296) -> ()  [unwired: 2 in, 2 out]
            n282 = property on="ReadFromFile" class="Bool (strict)"("Disabled"=w296) -> ()  [unwired: 2 in, 2 out]
            n283 = property on="Quit" class="Bool (strict)"("Disabled"=w296) -> ()  [unwired: 2 in, 2 out]
            n284 = property on="ConnectChannel" class="Bool (strict)"("Disabled"=w296) -> ()  [unwired: 2 in, 2 out]
            n285 = property on="DeleteChannel" class="Bool (strict)"("Disabled"=w296) -> ()  [unwired: 2 in, 2 out]
            n286 = property on="WriteToFile" class="Bool (strict)"("Disabled"=w296) -> ()  [unwired: 2 in, 2 out]
            n287 = property on="SetCurrentB" class="Bool (strict)"("Disabled"=w296) -> ()  [unwired: 2 in, 2 out]
            n288 = property on="SetOutputOnB" class="Bool (strict)"("Disabled"=w296) -> ()  [unwired: 2 in, 2 out]
            n289 = property on="SetVoltageB" class="Bool (strict)"("Disabled"=w296) -> ()  [unwired: 2 in, 2 out]
            n290 = property on="SetOutputOffB" class="Bool (strict)"("Disabled"=w296) -> ()  [unwired: 2 in, 2 out]
            n291 = property on="SetVoltageAll" class="Bool (strict)"("Disabled"=w296) -> ()  [unwired: 2 in, 2 out]
            n292 = property on="SetCurrentAll" class="Bool (strict)"("Disabled"=w296) -> ()  [unwired: 2 in, 2 out]
            n293 = property on="DisconnectAll" class="Bool (strict)"("Disabled"=w296) -> ()  [unwired: 2 in, 2 out]
          }
          frame #1 {
            w300 = FALSE ("OK Button")
            n294 = local write "DisconnectChannel"(w300) -> ()
            n295 = local read "Measure_VI"() -> (w302:refnum<vi>[])
            n296 = Index Array(array=w302, index=w299) -> (element=w301:refnum<vi>)
            n297 = invoke class="VI" method="Ctrl Val.Set"(reference=w301, "Control Name"="Connect", "Value"=w300) -> (error out=w298:errorcluster)  [unwired: 2 in, 4 out]
          }
          frame #2 {
            w305 = u8 0 ("Disabled")
            n298 = property on="AddChannel" class="Bool (strict)"("Disabled"=w305) -> ()  [unwired: 2 in, 2 out]
            n299 = property on="CurrentModulationB" class="Bool (strict)"("Disabled"=w305) -> ()  [unwired: 2 in, 2 out]
            n300 = property on="DisconnectChannel" class="Bool (strict)"("Disabled"=w305) -> ()  [unwired: 2 in, 2 out]
            n301 = property on="ConnectAll" class="Bool (strict)"("Disabled"=w305) -> ()  [unwired: 2 in, 2 out]
            n302 = property on="ReadFromFile" class="Bool (strict)"("Disabled"=w305) -> ()  [unwired: 2 in, 2 out]
            n303 = property on="ConnectChannel" class="Bool (strict)"("Disabled"=w305) -> ()  [unwired: 2 in, 2 out]
            n304 = property on="Quit" class="Bool (strict)"("Disabled"=w305) -> ()  [unwired: 2 in, 2 out]
            n305 = property on="DeleteChannel" class="Bool (strict)"("Disabled"=w305) -> ()  [unwired: 2 in, 2 out]
            n306 = property on="SetOutputOffB" class="Bool (strict)"("Disabled"=w305) -> ()  [unwired: 2 in, 2 out]
            n307 = property on="Set Output ON All" class="Bool (strict)"("Disabled"=w305) -> ()  [unwired: 2 in, 2 out]
            n308 = property on="SetVoltageAll" class="Bool (strict)"("Disabled"=w305) -> ()  [unwired: 2 in, 2 out]
            n309 = property on="SetCurrentAll" class="Bool (strict)"("Disabled"=w305) -> ()  [unwired: 2 in, 2 out]
            n310 = property on="DisconnectAll" class="Bool (strict)"("Disabled"=w305) -> ()  [unwired: 2 in, 2 out]
            n311 = property on="WriteToFile" class="Bool (strict)"("Disabled"=w305) -> ()  [unwired: 2 in, 2 out]
            n312 = property on="SetCurrentB" class="Bool (strict)"("Disabled"=w305) -> ()  [unwired: 2 in, 2 out]
            n313 = property on="SetOutputOnB" class="Bool (strict)"("Disabled"=w305) -> ()  [unwired: 2 in, 2 out]
            n314 = property on="SetVoltageB" class="Bool (strict)"("Disabled"=w305) -> ()  [unwired: 2 in, 2 out]
          }
        }
        n315 = Merge Errors(w293) -> (w291:errorcluster)
      }
      event "ConnectChannel": Value Change {
        n316 = event-data() -> ()  [unwired: 7 out]
        n317 = property on="List of channels" class="MCListbox (strict)"() -> ("Value"=w310:i32)  [unwired: 2 in, 2 out]
        n318 = flat-sequence {
          tunnel: w310 -> [w312]
          tunnel: [w312] -> w309
          tunnel: w309 -> [w317]
          tunnel: [w316] -> w307
          tunnel: [w329] -> w308
          tunnel: w307 -> [w329]
          frame #0 {
            w311 = u8 2 ("Disabled")
            n319 = property on="AddChannel" class="Bool (strict)"("Disabled"=w311) -> ()  [unwired: 2 in, 2 out]
            n320 = property on="Set Output ON All" class="Bool (strict)"("Disabled"=w311) -> ()  [unwired: 2 in, 2 out]
            n321 = property on="CurrentModulationB" class="Bool (strict)"("Disabled"=w311) -> ()  [unwired: 2 in, 2 out]
            n322 = property on="ConnectAll" class="Bool (strict)"("Disabled"=w311) -> ()  [unwired: 2 in, 2 out]
            n323 = property on="DisconnectChannel" class="Bool (strict)"("Disabled"=w311) -> ()  [unwired: 2 in, 2 out]
            n324 = property on="ReadFromFile" class="Bool (strict)"("Disabled"=w311) -> ()  [unwired: 2 in, 2 out]
            n325 = property on="Quit" class="Bool (strict)"("Disabled"=w311) -> ()  [unwired: 2 in, 2 out]
            n326 = property on="ConnectChannel" class="Bool (strict)"("Disabled"=w311) -> ()  [unwired: 2 in, 2 out]
            n327 = property on="DeleteChannel" class="Bool (strict)"("Disabled"=w311) -> ()  [unwired: 2 in, 2 out]
            n328 = property on="WriteToFile" class="Bool (strict)"("Disabled"=w311) -> ()  [unwired: 2 in, 2 out]
            n329 = property on="SetCurrentB" class="Bool (strict)"("Disabled"=w311) -> ()  [unwired: 2 in, 2 out]
            n330 = property on="SetOutputOnB" class="Bool (strict)"("Disabled"=w311) -> ()  [unwired: 2 in, 2 out]
            n331 = property on="SetVoltageB" class="Bool (strict)"("Disabled"=w311) -> ()  [unwired: 2 in, 2 out]
            n332 = property on="SetOutputOffB" class="Bool (strict)"("Disabled"=w311) -> ()  [unwired: 2 in, 2 out]
            n333 = property on="SetVoltageAll" class="Bool (strict)"("Disabled"=w311) -> ()  [unwired: 2 in, 2 out]
            n334 = property on="SetCurrentAll" class="Bool (strict)"("Disabled"=w311) -> ()  [unwired: 2 in, 2 out]
            n335 = property on="DisconnectAll" class="Bool (strict)"("Disabled"=w311) -> ()  [unwired: 2 in, 2 out]
          }
          frame #1 {
            n336 = local read "Measure_VI"() -> (w318:refnum<vi>[])
            n337 = Index Array(array=w318, index=w317) -> (element=w315:refnum<vi>)
            n338 = flat-sequence {
              tunnel: w315 -> [w320]
              tunnel: [w319] -> w313
              tunnel: [w323] -> w314
              tunnel: w313 -> [w323]
              tunnel: [w325] -> w316
              tunnel: w314 -> [w326]
              frame #0 {
                n339 = invoke class="VI" method="Ctrl Val.Set"(reference=w320, "Control Name"="Connect", "Value"=FALSE ("OK Button")) -> (reference out=w319:refnum<vi>)  [unwired: 2 in, 4 out]
              }
              frame #1 {
                n340 = Wait (ms)(milliseconds to wait=u32 1000) -> ()  [unwired: 1 out]
              }
              frame #2 {
                n341 = invoke class="VI" method="Ctrl Val.Set"(reference=w326, "Control Name"="Connect", "Value"=TRUE ("OK Button")) -> (error out=w325:errorcluster)  [unwired: 2 in, 4 out]
              }
            }
          }
          frame #2 {
            w330 = u8 0 ("Disabled")
            n342 = local write "ConnectChannel"(FALSE ("ConnectChannel")) -> ()
            n343 = property on="ConnectAll" class="Bool (strict)"("Disabled"=w330) -> ()  [unwired: 2 in, 2 out]
            n344 = property on="Set Output ON All" class="Bool (strict)"("Disabled"=w330) -> ()  [unwired: 2 in, 2 out]
            n345 = property on="AddChannel" class="Bool (strict)"("Disabled"=w330) -> ()  [unwired: 2 in, 2 out]
            n346 = property on="DisconnectChannel" class="Bool (strict)"("Disabled"=w330) -> ()  [unwired: 2 in, 2 out]
            n347 = property on="ReadFromFile" class="Bool (strict)"("Disabled"=w330) -> ()  [unwired: 2 in, 2 out]
            n348 = property on="ConnectChannel" class="Bool (strict)"("Disabled"=w330) -> ()  [unwired: 2 in, 2 out]
            n349 = property on="Quit" class="Bool (strict)"("Disabled"=w330) -> ()  [unwired: 2 in, 2 out]
            n350 = property on="DeleteChannel" class="Bool (strict)"("Disabled"=w330) -> ()  [unwired: 2 in, 2 out]
            n351 = property on="WriteToFile" class="Bool (strict)"("Disabled"=w330) -> ()  [unwired: 2 in, 2 out]
            n352 = property on="CurrentModulationB" class="Bool (strict)"("Disabled"=w330) -> ()  [unwired: 2 in, 2 out]
            n353 = property on="SetCurrentB" class="Bool (strict)"("Disabled"=w330) -> ()  [unwired: 2 in, 2 out]
            n354 = property on="SetOutputOnB" class="Bool (strict)"("Disabled"=w330) -> ()  [unwired: 2 in, 2 out]
            n355 = property on="SetVoltageB" class="Bool (strict)"("Disabled"=w330) -> ()  [unwired: 2 in, 2 out]
            n356 = property on="SetOutputOffB" class="Bool (strict)"("Disabled"=w330) -> ()  [unwired: 2 in, 2 out]
            n357 = property on="SetVoltageAll" class="Bool (strict)"("Disabled"=w330) -> ()  [unwired: 2 in, 2 out]
            n358 = property on="SetCurrentAll" class="Bool (strict)"("Disabled"=w330) -> ()  [unwired: 2 in, 2 out]
            n359 = property on="DisconnectAll" class="Bool (strict)"("Disabled"=w330) -> ()  [unwired: 2 in, 2 out]
          }
        }
        n360 = Merge Errors(w308) -> (w306:errorcluster)
      }
      event "ConnectAll": Value Change {
        n361 = event-data() -> ()  [unwired: 7 out]
        n362 = flat-sequence {
          tunnel: [w336] -> w333
          tunnel: [w345] -> w334
          tunnel: w333 -> [w345]
          frame #0 {
            w335 = u8 2 ("Disabled")
            n363 = property on="Quit" class="Bool (strict)"("Disabled"=w335) -> ()  [unwired: 2 in, 2 out]
            n364 = property on="ReadFromFile" class="Bool (strict)"("Disabled"=w335) -> ()  [unwired: 2 in, 2 out]
            n365 = property on="CurrentModulationB" class="Bool (strict)"("Disabled"=w335) -> ()  [unwired: 2 in, 2 out]
            n366 = property on="WriteToFile" class="Bool (strict)"("Disabled"=w335) -> ()  [unwired: 2 in, 2 out]
            n367 = property on="ConnectAll" class="Bool (strict)"("Disabled"=w335) -> ()  [unwired: 2 in, 2 out]
            n368 = property on="Set Output ON All" class="Bool (strict)"("Disabled"=w335) -> ()  [unwired: 2 in, 2 out]
            n369 = property on="SetOutputOffB" class="Bool (strict)"("Disabled"=w335) -> ()  [unwired: 2 in, 2 out]
            n370 = property on="AddChannel" class="Bool (strict)"("Disabled"=w335) -> ()  [unwired: 2 in, 2 out]
            n371 = property on="DisconnectChannel" class="Bool (strict)"("Disabled"=w335) -> ()  [unwired: 2 in, 2 out]
            n372 = property on="SetCurrentAll" class="Bool (strict)"("Disabled"=w335) -> ()  [unwired: 2 in, 2 out]
            n373 = property on="SetOutputOnB" class="Bool (strict)"("Disabled"=w335) -> ()  [unwired: 2 in, 2 out]
            n374 = property on="ConnectChannel" class="Bool (strict)"("Disabled"=w335) -> ()  [unwired: 2 in, 2 out]
            n375 = property on="DeleteChannel" class="Bool (strict)"("Disabled"=w335) -> ()  [unwired: 2 in, 2 out]
            n376 = property on="SetCurrentB" class="Bool (strict)"("Disabled"=w335) -> ()  [unwired: 2 in, 2 out]
            n377 = property on="SetVoltageB" class="Bool (strict)"("Disabled"=w335) -> ()  [unwired: 2 in, 2 out]
            n378 = property on="SetVoltageAll" class="Bool (strict)"("Disabled"=w335) -> ()  [unwired: 2 in, 2 out]
            n379 = property on="DisconnectAll" class="Bool (strict)"("Disabled"=w335) -> ()  [unwired: 2 in, 2 out]
          }
          frame #1 {
            n380 = local read "Measure_VI"() -> (w338:refnum<vi>[])
            n381 = Array Size(array=w338) -> (size(s)=w337:i32)
            n382 = for {
              N: w337 -> [_]
              tunnel: [w339] -> w336 mode=indexing
              i -> [w340]
              n383 = local read "Measure_VI"() -> (w343:refnum<vi>[])
              n384 = Index Array(array=w343, index=w340) -> (element=w342:refnum<vi>)
              n385 = invoke class="VI" method="Ctrl Val.Set"(reference=w342, "Control Name"="Connect", "Value"=TRUE ("OK Button")) -> (error out=w339:errorcluster)  [unwired: 2 in, 4 out]
            }
          }
          frame #2 {
            w346 = u8 0 ("Disabled")
            n386 = local write "ConnectAll"(FALSE ("ConnectChannel")) -> ()
            n387 = property on="Quit" class="Bool (strict)"("Disabled"=w346) -> ()  [unwired: 2 in, 2 out]
            n388 = property on="AddChannel" class="Bool (strict)"("Disabled"=w346) -> ()  [unwired: 2 in, 2 out]
            n389 = property on="DisconnectChannel" class="Bool (strict)"("Disabled"=w346) -> ()  [unwired: 2 in, 2 out]
            n390 = property on="ConnectAll" class="Bool (strict)"("Disabled"=w346) -> ()  [unwired: 2 in, 2 out]
            n391 = property on="Set Output ON All" class="Bool (strict)"("Disabled"=w346) -> ()  [unwired: 2 in, 2 out]
            n392 = property on="SetOutputOffB" class="Bool (strict)"("Disabled"=w346) -> ()  [unwired: 2 in, 2 out]
            n393 = property on="SetCurrentAll" class="Bool (strict)"("Disabled"=w346) -> ()  [unwired: 2 in, 2 out]
            n394 = property on="ConnectChannel" class="Bool (strict)"("Disabled"=w346) -> ()  [unwired: 2 in, 2 out]
            n395 = property on="SetVoltageAll" class="Bool (strict)"("Disabled"=w346) -> ()  [unwired: 2 in, 2 out]
            n396 = property on="SetOutputOnB" class="Bool (strict)"("Disabled"=w346) -> ()  [unwired: 2 in, 2 out]
            n397 = property on="CurrentModulationB" class="Bool (strict)"("Disabled"=w346) -> ()  [unwired: 2 in, 2 out]
            n398 = property on="DisconnectAll" class="Bool (strict)"("Disabled"=w346) -> ()  [unwired: 2 in, 2 out]
            n399 = property on="ReadFromFile" class="Bool (strict)"("Disabled"=w346) -> ()  [unwired: 2 in, 2 out]
            n400 = property on="WriteToFile" class="Bool (strict)"("Disabled"=w346) -> ()  [unwired: 2 in, 2 out]
            n401 = property on="SetCurrentB" class="Bool (strict)"("Disabled"=w346) -> ()  [unwired: 2 in, 2 out]
            n402 = property on="SetVoltageB" class="Bool (strict)"("Disabled"=w346) -> ()  [unwired: 2 in, 2 out]
            n403 = property on="DeleteChannel" class="Bool (strict)"("Disabled"=w346) -> ()  [unwired: 2 in, 2 out]
          }
        }
        n404 = Merge Errors(w334) -> (w332:errorcluster)
      }
      event "DisconnectAll": Value Change {
        n405 = event-data() -> ()  [unwired: 7 out]
        n406 = flat-sequence {
          tunnel: [w352] -> w350
          tunnel: [w361] -> w349
          tunnel: w350 -> [w361]
          frame #0 {
            w351 = u8 2 ("Disabled")
            n407 = property on="Quit" class="Bool (strict)"("Disabled"=w351) -> ()  [unwired: 2 in, 2 out]
            n408 = property on="ReadFromFile" class="Bool (strict)"("Disabled"=w351) -> ()  [unwired: 2 in, 2 out]
            n409 = property on="CurrentModulationB" class="Bool (strict)"("Disabled"=w351) -> ()  [unwired: 2 in, 2 out]
            n410 = property on="ConnectAll" class="Bool (strict)"("Disabled"=w351) -> ()  [unwired: 2 in, 2 out]
            n411 = property on="ConnectChannel" class="Bool (strict)"("Disabled"=w351) -> ()  [unwired: 2 in, 2 out]
            n412 = property on="AddChannel" class="Bool (strict)"("Disabled"=w351) -> ()  [unwired: 2 in, 2 out]
            n413 = property on="DisconnectChannel" class="Bool (strict)"("Disabled"=w351) -> ()  [unwired: 2 in, 2 out]
            n414 = property on="Set Output ON All" class="Bool (strict)"("Disabled"=w351) -> ()  [unwired: 2 in, 2 out]
            n415 = property on="WriteToFile" class="Bool (strict)"("Disabled"=w351) -> ()  [unwired: 2 in, 2 out]
            n416 = property on="SetOutputOffB" class="Bool (strict)"("Disabled"=w351) -> ()  [unwired: 2 in, 2 out]
            n417 = property on="SetCurrentAll" class="Bool (strict)"("Disabled"=w351) -> ()  [unwired: 2 in, 2 out]
            n418 = property on="SetOutputOnB" class="Bool (strict)"("Disabled"=w351) -> ()  [unwired: 2 in, 2 out]
            n419 = property on="DeleteChannel" class="Bool (strict)"("Disabled"=w351) -> ()  [unwired: 2 in, 2 out]
            n420 = property on="SetCurrentB" class="Bool (strict)"("Disabled"=w351) -> ()  [unwired: 2 in, 2 out]
            n421 = property on="SetVoltageB" class="Bool (strict)"("Disabled"=w351) -> ()  [unwired: 2 in, 2 out]
            n422 = property on="SetVoltageAll" class="Bool (strict)"("Disabled"=w351) -> ()  [unwired: 2 in, 2 out]
            n423 = property on="DisconnectAll" class="Bool (strict)"("Disabled"=w351) -> ()  [unwired: 2 in, 2 out]
          }
          frame #1 {
            n424 = local read "Measure_VI"() -> (w354:refnum<vi>[])
            n425 = Array Size(array=w354) -> (size(s)=w353:i32)
            n426 = for {
              N: w353 -> [_]
              tunnel: [w355] -> w352 mode=indexing
              i -> [w356]
              n427 = local read "Measure_VI"() -> (w359:refnum<vi>[])
              n428 = Index Array(array=w359, index=w356) -> (element=w358:refnum<vi>)
              n429 = invoke class="VI" method="Ctrl Val.Set"(reference=w358, "Control Name"="Connect", "Value"=FALSE ("OK Button")) -> (error out=w355:errorcluster)  [unwired: 2 in, 4 out]
            }
          }
          frame #2 {
            w362 = u8 0 ("Disabled")
            n430 = local write "DisconnectAll"(FALSE ("ConnectChannel")) -> ()
            n431 = property on="Quit" class="Bool (strict)"("Disabled"=w362) -> ()  [unwired: 2 in, 2 out]
            n432 = property on="ConnectAll" class="Bool (strict)"("Disabled"=w362) -> ()  [unwired: 2 in, 2 out]
            n433 = property on="ConnectChannel" class="Bool (strict)"("Disabled"=w362) -> ()  [unwired: 2 in, 2 out]
            n434 = property on="AddChannel" class="Bool (strict)"("Disabled"=w362) -> ()  [unwired: 2 in, 2 out]
            n435 = property on="DisconnectChannel" class="Bool (strict)"("Disabled"=w362) -> ()  [unwired: 2 in, 2 out]
            n436 = property on="ReadFromFile" class="Bool (strict)"("Disabled"=w362) -> ()  [unwired: 2 in, 2 out]
            n437 = property on="Set Output ON All" class="Bool (strict)"("Disabled"=w362) -> ()  [unwired: 2 in, 2 out]
            n438 = property on="WriteToFile" class="Bool (strict)"("Disabled"=w362) -> ()  [unwired: 2 in, 2 out]
            n439 = property on="SetOutputOnB" class="Bool (strict)"("Disabled"=w362) -> ()  [unwired: 2 in, 2 out]
            n440 = property on="CurrentModulationB" class="Bool (strict)"("Disabled"=w362) -> ()  [unwired: 2 in, 2 out]
            n441 = property on="SetCurrentB" class="Bool (strict)"("Disabled"=w362) -> ()  [unwired: 2 in, 2 out]
            n442 = property on="SetVoltageB" class="Bool (strict)"("Disabled"=w362) -> ()  [unwired: 2 in, 2 out]
            n443 = property on="SetVoltageAll" class="Bool (strict)"("Disabled"=w362) -> ()  [unwired: 2 in, 2 out]
            n444 = property on="DisconnectAll" class="Bool (strict)"("Disabled"=w362) -> ()  [unwired: 2 in, 2 out]
            n445 = property on="DeleteChannel" class="Bool (strict)"("Disabled"=w362) -> ()  [unwired: 2 in, 2 out]
            n446 = property on="SetOutputOffB" class="Bool (strict)"("Disabled"=w362) -> ()  [unwired: 2 in, 2 out]
            n447 = property on="SetCurrentAll" class="Bool (strict)"("Disabled"=w362) -> ()  [unwired: 2 in, 2 out]
          }
        }
        n448 = Merge Errors(w349) -> (w348:errorcluster)
      }
      event "SetVoltageB": Value Change {
        n449 = event-data() -> ()  [unwired: 7 out]
        n450 = local write "SetVoltageB"(FALSE ("ConnectChannel")) -> ()
        n451 = flat-sequence {
          tunnel: [w370] -> w366
          tunnel: [w379] -> w365
          tunnel: w366 -> [w379]
          frame #0 {
            w368 = u8 2 ("Disabled")
            n452 = property on="Quit" class="Bool (strict)"("Disabled"=w368) -> ()  [unwired: 2 in, 2 out]
            n453 = property on="AddChannel" class="Bool (strict)"("Disabled"=w368) -> ()  [unwired: 2 in, 2 out]
            n454 = property on="Set Output ON All" class="Bool (strict)"("Disabled"=w368) -> ()  [unwired: 2 in, 2 out]
            n455 = property on="CurrentModulationB" class="Bool (strict)"("Disabled"=w368) -> ()  [unwired: 2 in, 2 out]
            n456 = property on="ConnectAll" class="Bool (strict)"("Disabled"=w368) -> ()  [unwired: 2 in, 2 out]
            n457 = property on="DisconnectChannel" class="Bool (strict)"("Disabled"=w368) -> ()  [unwired: 2 in, 2 out]
            n458 = property on="ReadFromFile" class="Bool (strict)"("Disabled"=w368) -> ()  [unwired: 2 in, 2 out]
            n459 = property on="ConnectChannel" class="Bool (strict)"("Disabled"=w368) -> ()  [unwired: 2 in, 2 out]
            n460 = property on="DeleteChannel" class="Bool (strict)"("Disabled"=w368) -> ()  [unwired: 2 in, 2 out]
            n461 = property on="WriteToFile" class="Bool (strict)"("Disabled"=w368) -> ()  [unwired: 2 in, 2 out]
            n462 = property on="SetCurrentB" class="Bool (strict)"("Disabled"=w368) -> ()  [unwired: 2 in, 2 out]
            n463 = property on="SetOutputOnB" class="Bool (strict)"("Disabled"=w368) -> ()  [unwired: 2 in, 2 out]
            n464 = property on="SetVoltageB" class="Bool (strict)"("Disabled"=w368) -> ()  [unwired: 2 in, 2 out]
            n465 = property on="SetOutputOffB" class="Bool (strict)"("Disabled"=w368) -> ()  [unwired: 2 in, 2 out]
            n466 = property on="SetVoltageAll" class="Bool (strict)"("Disabled"=w368) -> ()  [unwired: 2 in, 2 out]
            n467 = property on="SetCurrentAll" class="Bool (strict)"("Disabled"=w368) -> ()  [unwired: 2 in, 2 out]
            n468 = property on="DisconnectAll" class="Bool (strict)"("Disabled"=w368) -> ()  [unwired: 2 in, 2 out]
          }
          frame #1 {
            n469 = property on="List of channels" class="MCListbox (strict)"() -> ("Value"=w369:i32)  [unwired: 2 in, 2 out]
            n470 = local read "Measure_VI"() -> (w377:refnum<vi>[])
            n471 = local read "SetVoltage"() -> (w375:dbl)
            n472 = Index Array(array=w377, index=w369) -> (element=w376:refnum<vi>)
            n473 = invoke class="VI" method="Ctrl Val.Set"(reference=w376, "Control Name"="SetVoltage", "Value"=w375) -> (reference out=w372:refnum<vi>, error out=w371:errorcluster)  [unwired: 2 in, 3 out]
            n474 = invoke class="VI" method="Ctrl Val.Set"(reference=w372, error in=w371, "Control Name"="NeedToSetVoltage", "Value"=TRUE ("ConnectChannel")) -> (error out=w370:errorcluster)  [unwired: 1 in, 4 out]
          }
          frame #2 {
            w380 = u8 0 ("Disabled")
            n475 = property on="Quit" class="Bool (strict)"("Disabled"=w380) -> ()  [unwired: 2 in, 2 out]
            n476 = property on="ConnectAll" class="Bool (strict)"("Disabled"=w380) -> ()  [unwired: 2 in, 2 out]
            n477 = property on="Set Output ON All" class="Bool (strict)"("Disabled"=w380) -> ()  [unwired: 2 in, 2 out]
            n478 = property on="AddChannel" class="Bool (strict)"("Disabled"=w380) -> ()  [unwired: 2 in, 2 out]
            n479 = property on="CurrentModulationB" class="Bool (strict)"("Disabled"=w380) -> ()  [unwired: 2 in, 2 out]
            n480 = property on="DisconnectChannel" class="Bool (strict)"("Disabled"=w380) -> ()  [unwired: 2 in, 2 out]
            n481 = property on="ReadFromFile" class="Bool (strict)"("Disabled"=w380) -> ()  [unwired: 2 in, 2 out]
            n482 = property on="ConnectChannel" class="Bool (strict)"("Disabled"=w380) -> ()  [unwired: 2 in, 2 out]
            n483 = property on="DeleteChannel" class="Bool (strict)"("Disabled"=w380) -> ()  [unwired: 2 in, 2 out]
            n484 = property on="SetVoltageAll" class="Bool (strict)"("Disabled"=w380) -> ()  [unwired: 2 in, 2 out]
            n485 = property on="SetCurrentAll" class="Bool (strict)"("Disabled"=w380) -> ()  [unwired: 2 in, 2 out]
            n486 = property on="DisconnectAll" class="Bool (strict)"("Disabled"=w380) -> ()  [unwired: 2 in, 2 out]
            n487 = property on="WriteToFile" class="Bool (strict)"("Disabled"=w380) -> ()  [unwired: 2 in, 2 out]
            n488 = property on="SetCurrentB" class="Bool (strict)"("Disabled"=w380) -> ()  [unwired: 2 in, 2 out]
            n489 = property on="SetOutputOnB" class="Bool (strict)"("Disabled"=w380) -> ()  [unwired: 2 in, 2 out]
            n490 = property on="SetVoltageB" class="Bool (strict)"("Disabled"=w380) -> ()  [unwired: 2 in, 2 out]
            n491 = property on="SetOutputOffB" class="Bool (strict)"("Disabled"=w380) -> ()  [unwired: 2 in, 2 out]
          }
        }
        n492 = Merge Errors(w365) -> (w364:errorcluster)
      }
      event "SetOutputOnB": Value Change {
        n493 = event-data() -> ()  [unwired: 2 out]
        n494 = property on="List of channels" class="MCListbox (strict)"() -> ("Value"=w384:i32)  [unwired: 2 in, 2 out]
        n495 = flat-sequence {
          tunnel: w384 -> [w386]
          tunnel: [w386] -> w383
          tunnel: w383 -> [w393]
          tunnel: [w388] -> w382
          tunnel: [w398] -> w381
          tunnel: w382 -> [w398]
          frame #0 {
            w385 = u8 2 ("Disabled")
            n496 = property on="ConnectAll" class="Bool (strict)"("Disabled"=w385) -> ()  [unwired: 2 in, 2 out]
            n497 = property on="Set Output ON All" class="Bool (strict)"("Disabled"=w385) -> ()  [unwired: 2 in, 2 out]
            n498 = property on="AddChannel" class="Bool (strict)"("Disabled"=w385) -> ()  [unwired: 2 in, 2 out]
            n499 = property on="CurrentModulationB" class="Bool (strict)"("Disabled"=w385) -> ()  [unwired: 2 in, 2 out]
            n500 = property on="DisconnectChannel" class="Bool (strict)"("Disabled"=w385) -> ()  [unwired: 2 in, 2 out]
            n501 = property on="ReadFromFile" class="Bool (strict)"("Disabled"=w385) -> ()  [unwired: 2 in, 2 out]
            n502 = property on="Quit" class="Bool (strict)"("Disabled"=w385) -> ()  [unwired: 2 in, 2 out]
            n503 = property on="ConnectChannel" class="Bool (strict)"("Disabled"=w385) -> ()  [unwired: 2 in, 2 out]
            n504 = property on="DeleteChannel" class="Bool (strict)"("Disabled"=w385) -> ()  [unwired: 2 in, 2 out]
            n505 = property on="WriteToFile" class="Bool (strict)"("Disabled"=w385) -> ()  [unwired: 2 in, 2 out]
            n506 = property on="SetCurrentB" class="Bool (strict)"("Disabled"=w385) -> ()  [unwired: 2 in, 2 out]
            n507 = property on="SetOutputOnB" class="Bool (strict)"("Disabled"=w385) -> ()  [unwired: 2 in, 2 out]
            n508 = property on="SetVoltageB" class="Bool (strict)"("Disabled"=w385) -> ()  [unwired: 2 in, 2 out]
            n509 = property on="SetOutputOffB" class="Bool (strict)"("Disabled"=w385) -> ()  [unwired: 2 in, 2 out]
            n510 = property on="SetVoltageAll" class="Bool (strict)"("Disabled"=w385) -> ()  [unwired: 2 in, 2 out]
            n511 = property on="SetCurrentAll" class="Bool (strict)"("Disabled"=w385) -> ()  [unwired: 2 in, 2 out]
            n512 = property on="DisconnectAll" class="Bool (strict)"("Disabled"=w385) -> ()  [unwired: 2 in, 2 out]
          }
          frame #1 {
            n513 = local write "SetOutputOnB"(FALSE ("ConnectChannel")) -> ()
            n514 = local read "Measure_VI"() -> (w396:refnum<vi>[])
            n515 = Index Array(array=w396, index=w393) -> (element=w395:refnum<vi>)
            n516 = invoke class="VI" method="Ctrl Val.Set"(reference=w395, "Control Name"="SetOutput", "Value"=TRUE ("ConnectChannel")) -> (reference out=w390:refnum<vi>, error out=w389:errorcluster)  [unwired: 2 in, 3 out]
            n517 = invoke class="VI" method="Ctrl Val.Set"(reference=w390, error in=w389, "Control Name"="NeedToSetOutput", "Value"=TRUE ("ConnectChannel")) -> (error out=w388:errorcluster)  [unwired: 1 in, 4 out]
          }
          frame #2 {
            w399 = u8 0 ("Disabled")
            n518 = property on="ConnectAll" class="Bool (strict)"("Disabled"=w399) -> ()  [unwired: 2 in, 2 out]
            n519 = property on="Set Output ON All" class="Bool (strict)"("Disabled"=w399) -> ()  [unwired: 2 in, 2 out]
            n520 = property on="AddChannel" class="Bool (strict)"("Disabled"=w399) -> ()  [unwired: 2 in, 2 out]
            n521 = property on="DisconnectChannel" class="Bool (strict)"("Disabled"=w399) -> ()  [unwired: 2 in, 2 out]
            n522 = property on="ReadFromFile" class="Bool (strict)"("Disabled"=w399) -> ()  [unwired: 2 in, 2 out]
            n523 = property on="ConnectChannel" class="Bool (strict)"("Disabled"=w399) -> ()  [unwired: 2 in, 2 out]
            n524 = property on="Quit" class="Bool (strict)"("Disabled"=w399) -> ()  [unwired: 2 in, 2 out]
            n525 = property on="DeleteChannel" class="Bool (strict)"("Disabled"=w399) -> ()  [unwired: 2 in, 2 out]
            n526 = property on="SetOutputOffB" class="Bool (strict)"("Disabled"=w399) -> ()  [unwired: 2 in, 2 out]
            n527 = property on="CurrentModulationB" class="Bool (strict)"("Disabled"=w399) -> ()  [unwired: 2 in, 2 out]
            n528 = property on="SetVoltageAll" class="Bool (strict)"("Disabled"=w399) -> ()  [unwired: 2 in, 2 out]
            n529 = property on="SetCurrentAll" class="Bool (strict)"("Disabled"=w399) -> ()  [unwired: 2 in, 2 out]
            n530 = property on="DisconnectAll" class="Bool (strict)"("Disabled"=w399) -> ()  [unwired: 2 in, 2 out]
            n531 = property on="WriteToFile" class="Bool (strict)"("Disabled"=w399) -> ()  [unwired: 2 in, 2 out]
            n532 = property on="SetCurrentB" class="Bool (strict)"("Disabled"=w399) -> ()  [unwired: 2 in, 2 out]
            n533 = property on="SetOutputOnB" class="Bool (strict)"("Disabled"=w399) -> ()  [unwired: 2 in, 2 out]
            n534 = property on="SetVoltageB" class="Bool (strict)"("Disabled"=w399) -> ()  [unwired: 2 in, 2 out]
          }
        }
      }
      event "Set Output ON All": Value Change {
        n535 = event-data() -> ("NewVal"=w400:bool)  [unwired: 1 out]
        n536 = flat-sequence {
          tunnel: [w405] -> w401
          tunnel: w400 -> [w405]
          tunnel: [w410] -> w403
          tunnel: w401 -> [w407]
          tunnel: [w421] -> w404
          tunnel: w403 -> [w421]
          frame #0 {
            w406 = u8 2 ("Disabled")
            n537 = property on="Quit" class="Bool (strict)"("Disabled"=w406) -> ()  [unwired: 2 in, 2 out]
            n538 = property on="AddChannel" class="Bool (strict)"("Disabled"=w406) -> ()  [unwired: 2 in, 2 out]
            n539 = property on="CurrentModulationB" class="Bool (strict)"("Disabled"=w406) -> ()  [unwired: 2 in, 2 out]
            n540 = property on="DisconnectChannel" class="Bool (strict)"("Disabled"=w406) -> ()  [unwired: 2 in, 2 out]
            n541 = property on="ConnectAll" class="Bool (strict)"("Disabled"=w406) -> ()  [unwired: 2 in, 2 out]
            n542 = property on="ReadFromFile" class="Bool (strict)"("Disabled"=w406) -> ()  [unwired: 2 in, 2 out]
            n543 = property on="ConnectChannel" class="Bool (strict)"("Disabled"=w406) -> ()  [unwired: 2 in, 2 out]
            n544 = property on="DeleteChannel" class="Bool (strict)"("Disabled"=w406) -> ()  [unwired: 2 in, 2 out]
            n545 = property on="WriteToFile" class="Bool (strict)"("Disabled"=w406) -> ()  [unwired: 2 in, 2 out]
            n546 = property on="SetCurrentB" class="Bool (strict)"("Disabled"=w406) -> ()  [unwired: 2 in, 2 out]
            n547 = property on="SetOutputOnB" class="Bool (strict)"("Disabled"=w406) -> ()  [unwired: 2 in, 2 out]
            n548 = property on="SetVoltageB" class="Bool (strict)"("Disabled"=w406) -> ()  [unwired: 2 in, 2 out]
            n549 = property on="SetOutputOffB" class="Bool (strict)"("Disabled"=w406) -> ()  [unwired: 2 in, 2 out]
            n550 = property on="SetVoltageAll" class="Bool (strict)"("Disabled"=w406) -> ()  [unwired: 2 in, 2 out]
            n551 = property on="SetCurrentAll" class="Bool (strict)"("Disabled"=w406) -> ()  [unwired: 2 in, 2 out]
            n552 = property on="DisconnectAll" class="Bool (strict)"("Disabled"=w406) -> ()  [unwired: 2 in, 2 out]
          }
          frame #1 {
            n553 = local read "Measure_VI"() -> (w409:refnum<vi>[])
            n554 = Array Size(array=w409) -> (size(s)=w408:i32)
            n555 = for {
              N: w408 -> [_]
              tunnel: [w412] -> w410 mode=indexing
              tunnel: w407 -> [w411]
              i -> [w414]
              n556 = local read "Measure_VI"() -> (w419:refnum<vi>[])
              n557 = Index Array(array=w419, index=w414) -> (element=w418:refnum<vi>)
              n558 = invoke class="VI" method="Ctrl Val.Set"(reference=w418, "Control Name"="SetOutput", "Value"=w411) -> (reference out=w415:refnum<vi>, error out=w413:errorcluster)  [unwired: 2 in, 3 out]
              n559 = invoke class="VI" method="Ctrl Val.Set"(reference=w415, error in=w413, "Control Name"="NeedToSetOutput", "Value"=TRUE ("ConnectChannel")) -> (error out=w412:errorcluster)  [unwired: 1 in, 4 out]
            }
          }
          frame #2 {
            w422 = u8 0 ("Disabled")
            n560 = disable-structure shown="Disabled" {
              frame Disabled {
                n561 = local write "Set Output ON All"(FALSE ("ConnectChannel")) -> ()
              }
              frame Enabled {
              }
            }
            n562 = property on="Quit" class="Bool (strict)"("Disabled"=w422) -> ()  [unwired: 2 in, 2 out]
            n563 = property on="ConnectAll" class="Bool (strict)"("Disabled"=w422) -> ()  [unwired: 2 in, 2 out]
            n564 = property on="Set Output ON All" class="Bool (strict)"("Disabled"=w422) -> ()  [unwired: 2 in, 2 out]
            n565 = property on="AddChannel" class="Bool (strict)"("Disabled"=w422) -> ()  [unwired: 2 in, 2 out]
            n566 = property on="DisconnectChannel" class="Bool (strict)"("Disabled"=w422) -> ()  [unwired: 2 in, 2 out]
            n567 = property on="ReadFromFile" class="Bool (strict)"("Disabled"=w422) -> ()  [unwired: 2 in, 2 out]
            n568 = property on="ConnectChannel" class="Bool (strict)"("Disabled"=w422) -> ()  [unwired: 2 in, 2 out]
            n569 = property on="DeleteChannel" class="Bool (strict)"("Disabled"=w422) -> ()  [unwired: 2 in, 2 out]
            n570 = property on="SetVoltageB" class="Bool (strict)"("Disabled"=w422) -> ()  [unwired: 2 in, 2 out]
            n571 = property on="CurrentModulationB" class="Bool (strict)"("Disabled"=w422) -> ()  [unwired: 2 in, 2 out]
            n572 = property on="SetOutputOffB" class="Bool (strict)"("Disabled"=w422) -> ()  [unwired: 2 in, 2 out]
            n573 = property on="SetVoltageAll" class="Bool (strict)"("Disabled"=w422) -> ()  [unwired: 2 in, 2 out]
            n574 = property on="SetCurrentAll" class="Bool (strict)"("Disabled"=w422) -> ()  [unwired: 2 in, 2 out]
            n575 = property on="DisconnectAll" class="Bool (strict)"("Disabled"=w422) -> ()  [unwired: 2 in, 2 out]
            n576 = property on="WriteToFile" class="Bool (strict)"("Disabled"=w422) -> ()  [unwired: 2 in, 2 out]
            n577 = property on="SetCurrentB" class="Bool (strict)"("Disabled"=w422) -> ()  [unwired: 2 in, 2 out]
            n578 = property on="SetOutputOnB" class="Bool (strict)"("Disabled"=w422) -> ()  [unwired: 2 in, 2 out]
          }
        }
        n579 = Merge Errors(w404) -> (w402:errorcluster)
      }
      event "SetOutputOffB": Value Change {
        n580 = event-data() -> ()  [unwired: 7 out]
        n581 = local write "SetOutputOffB"(FALSE ("ConnectChannel")) -> ()
        n582 = property on="List of channels" class="MCListbox (strict)"() -> ("Value"=w428:i32)  [unwired: 2 in, 2 out]
        n583 = flat-sequence {
          tunnel: w428 -> [w430]
          tunnel: [w430] -> w427
          tunnel: w427 -> [w437]
          tunnel: [w431] -> w424
          tunnel: [w441] -> w425
          tunnel: w424 -> [w441]
          frame #0 {
            w429 = u8 2 ("Disabled")
            n584 = property on="ConnectAll" class="Bool (strict)"("Disabled"=w429) -> ()  [unwired: 2 in, 2 out]
            n585 = property on="Set Output ON All" class="Bool (strict)"("Disabled"=w429) -> ()  [unwired: 2 in, 2 out]
            n586 = property on="AddChannel" class="Bool (strict)"("Disabled"=w429) -> ()  [unwired: 2 in, 2 out]
            n587 = property on="CurrentModulationB" class="Bool (strict)"("Disabled"=w429) -> ()  [unwired: 2 in, 2 out]
            n588 = property on="DisconnectChannel" class="Bool (strict)"("Disabled"=w429) -> ()  [unwired: 2 in, 2 out]
            n589 = property on="ReadFromFile" class="Bool (strict)"("Disabled"=w429) -> ()  [unwired: 2 in, 2 out]
            n590 = property on="Quit" class="Bool (strict)"("Disabled"=w429) -> ()  [unwired: 2 in, 2 out]
            n591 = property on="ConnectChannel" class="Bool (strict)"("Disabled"=w429) -> ()  [unwired: 2 in, 2 out]
            n592 = property on="DeleteChannel" class="Bool (strict)"("Disabled"=w429) -> ()  [unwired: 2 in, 2 out]
            n593 = property on="WriteToFile" class="Bool (strict)"("Disabled"=w429) -> ()  [unwired: 2 in, 2 out]
            n594 = property on="SetCurrentB" class="Bool (strict)"("Disabled"=w429) -> ()  [unwired: 2 in, 2 out]
            n595 = property on="SetOutputOnB" class="Bool (strict)"("Disabled"=w429) -> ()  [unwired: 2 in, 2 out]
            n596 = property on="SetVoltageB" class="Bool (strict)"("Disabled"=w429) -> ()  [unwired: 2 in, 2 out]
            n597 = property on="SetOutputOffB" class="Bool (strict)"("Disabled"=w429) -> ()  [unwired: 2 in, 2 out]
            n598 = property on="SetVoltageAll" class="Bool (strict)"("Disabled"=w429) -> ()  [unwired: 2 in, 2 out]
            n599 = property on="SetCurrentAll" class="Bool (strict)"("Disabled"=w429) -> ()  [unwired: 2 in, 2 out]
            n600 = property on="DisconnectAll" class="Bool (strict)"("Disabled"=w429) -> ()  [unwired: 2 in, 2 out]
          }
          frame #1 {
            n601 = local read "Measure_VI"() -> (w439:refnum<vi>[])
            n602 = Index Array(array=w439, index=w437) -> (element=w438:refnum<vi>)
            n603 = invoke class="VI" method="Ctrl Val.Set"(reference=w438, "Control Name"="SetOutput", "Value"=FALSE ("ConnectChannel")) -> (reference out=w434:refnum<vi>, error out=w432:errorcluster)  [unwired: 2 in, 3 out]
            n604 = invoke class="VI" method="Ctrl Val.Set"(reference=w434, error in=w432, "Control Name"="NeedToSetOutput", "Value"=TRUE ("ConnectChannel")) -> (error out=w431:errorcluster)  [unwired: 1 in, 4 out]
          }
          frame #2 {
            w442 = u8 0 ("Disabled")
            n605 = property on="ConnectAll" class="Bool (strict)"("Disabled"=w442) -> ()  [unwired: 2 in, 2 out]
            n606 = property on="Set Output ON All" class="Bool (strict)"("Disabled"=w442) -> ()  [unwired: 2 in, 2 out]
            n607 = property on="AddChannel" class="Bool (strict)"("Disabled"=w442) -> ()  [unwired: 2 in, 2 out]
            n608 = property on="CurrentModulationB" class="Bool (strict)"("Disabled"=w442) -> ()  [unwired: 2 in, 2 out]
            n609 = property on="DisconnectChannel" class="Bool (strict)"("Disabled"=w442) -> ()  [unwired: 2 in, 2 out]
            n610 = property on="ReadFromFile" class="Bool (strict)"("Disabled"=w442) -> ()  [unwired: 2 in, 2 out]
            n611 = property on="ConnectChannel" class="Bool (strict)"("Disabled"=w442) -> ()  [unwired: 2 in, 2 out]
            n612 = property on="Quit" class="Bool (strict)"("Disabled"=w442) -> ()  [unwired: 2 in, 2 out]
            n613 = property on="DeleteChannel" class="Bool (strict)"("Disabled"=w442) -> ()  [unwired: 2 in, 2 out]
            n614 = property on="SetOutputOffB" class="Bool (strict)"("Disabled"=w442) -> ()  [unwired: 2 in, 2 out]
            n615 = property on="SetVoltageAll" class="Bool (strict)"("Disabled"=w442) -> ()  [unwired: 2 in, 2 out]
            n616 = property on="SetCurrentAll" class="Bool (strict)"("Disabled"=w442) -> ()  [unwired: 2 in, 2 out]
            n617 = property on="DisconnectAll" class="Bool (strict)"("Disabled"=w442) -> ()  [unwired: 2 in, 2 out]
            n618 = property on="WriteToFile" class="Bool (strict)"("Disabled"=w442) -> ()  [unwired: 2 in, 2 out]
            n619 = property on="SetCurrentB" class="Bool (strict)"("Disabled"=w442) -> ()  [unwired: 2 in, 2 out]
            n620 = property on="SetOutputOnB" class="Bool (strict)"("Disabled"=w442) -> ()  [unwired: 2 in, 2 out]
            n621 = property on="SetVoltageB" class="Bool (strict)"("Disabled"=w442) -> ()  [unwired: 2 in, 2 out]
          }
        }
      }
      event "WriteToFile": Value Change {
        n622 = event-data() -> ()  [unwired: 7 out]
        n623 = local read "ADRESS"() -> (w447:string[])
        n624 = Array Size(array=w447) -> (size(s)=w446:i32)
        n625 = flat-sequence {
          tunnel: w446 -> [w456]
          tunnel: [w448] -> w444
          tunnel: [w489] -> w445
          tunnel: w444 -> [w489]
          frame #0 {
            n626 = Number To Decimal String(number=w456) -> (decimal integer string=w451:string)  [unwired: 1 out]
            n627 = Write to Text File(text=w451) -> (refnum out=w450:refnum<file>, cancelled=w449:bool, error out=w452:errorcluster)  [unwired: 1 in, 2 out]
            n628 = Write to Text File(file (use dialog)=w450, text="\nИМЯ  АДРЕС  ТОК  НАПРЯЖЕНИЕ", error in=w452) -> (refnum out=w453:refnum<file>, error out=w454:errorcluster)  [unwired: 2 out]
            n629 = for {
              N: w456 -> [_]
              tunnel: w449 -> [w466]
              tunnel: w454 -> [w461]
              tunnel: w453 -> [w468]
              tunnel: [w459] -> w448 mode=indexing
              i -> [w467]
              w472 = "" ("Control Name")
              w478 = "\t"
              n630 = local read "Measure_VI"() -> (w476:refnum<vi>[])
              n631 = Index Array(array=w476, index=w467) -> (element=w475:refnum<vi>)
              n632 = invoke class="VI" method="Ctrl Val.Get"(reference=w475, "Control Name"="SetVoltageStr") -> (reference out=w470:refnum<vi>, error out=w463:errorcluster, "Get Control Value Variant"=w477:variant)  [unwired: 2 in, 1 out]
              n633 = invoke class="VI" method="Ctrl Val.Get"(reference=w470, error in=w463, "Control Name"="SetCurrentStr") -> (error out=w462:errorcluster, "Get Control Value Variant"=w473:variant)  [unwired: 1 in, 2 out]
              n634 = local read "ADRESS"() -> (w483:string[])
              n635 = local read "NAME"() -> (w481:string[])
              n636 = Index Array(array=w481, index=w467) -> (element=w479:string)
              n637 = Index Array(array=w483, index=w467) -> (element=w482:string)
              n638 = Variant To Data(type=w472, Variant=w473) -> (data=w457:string, error out=w465:errorcluster)  [unwired: 1 in]
              n639 = Variant To Data(type=w472, Variant=w477) -> (data=w458:string, error out=w464:errorcluster)  [unwired: 1 in]
              n640 = Merge Errors(w462, w465, w464, w461) -> (w460:errorcluster)
              n641 = Concatenate Strings("\r\n", w479, w478, w482, w478, w458, w478, w457) -> (w469:string)
              n642 = case shown="False" w466 {
                tunnel: w468 -> [w486 _]
                tunnel: w469 -> [w487 _]
                tunnel: w460 -> [w485 w488]
                tunnel: [w484 w488] -> w459
                frame False {
                  n643 = Write to Text File(file (use dialog)=w486, text=w487, error in=w485) -> (error out=w484:errorcluster)  [unwired: 3 out]
                }
                frame True {
                }
              }
            }
          }
          frame #1 {
            n644 = local write "WriteToFile"(FALSE ("ConnectChannel")) -> ()
          }
        }
        n645 = Merge Errors(w445) -> (w443:errorcluster)
      }
      event "ReadFromFile": Value Change {
        n646 = event-data() -> ()  [unwired: 2 out]
        n647 = Read from Text File(count=100) -> (text=w497:string[], cancelled=w496:bool, error out=w495:errorcluster)  [unwired: 1 in, 3 out]
        n648 = local read "ReadFromFile"() -> (w493:bool)
        n649 = Not(x=w496) -> (.not. x?=w492:bool)
        n650 = And(x=w493, y=w492) -> (x .and. y?=w491:bool)
        n651 = case shown="True" w491 {
          tunnel: w497 -> [_ w501]
          tunnel: w495 -> [w499 w503]
          tunnel: [w499 w502] -> w494
          frame False {
            n652 = local write "ReadFromFile"(FALSE ("ConnectChannel")) -> ()
          }
          frame True {
            n653 = flat-sequence {
              tunnel: w503 -> [w510]
              tunnel: [w509] -> w505
              tunnel: w505 -> [w524]
              tunnel: [w524] -> w504
              tunnel: w504 -> [_]
              tunnel: [w534] -> w507
              tunnel: w501 -> [w533]
              tunnel: w507 -> [w568]
              tunnel: [w568] -> w506
              frame #0 {
                w508 = u8 2 ("Disabled")
                n654 = disable-structure shown="Enabled" {
                  disable-tunnel: w510 -> [w513 w522]
                  disable-tunnel: [w512 w522] -> w509
                  frame Disabled {
                    n655 = local read "Measure_VI"() -> (w514:refnum<vi>[])
                    n656 = Array Size(array=w514) -> (size(s)=w511:i32)
                    n657 = for {
                      N: w511 -> [_]
                      tunnel: w514 -> [w518]
                      tunnel: w513 -> [w516]
                      tunnel: [w515] -> w512 mode=indexing
                      i -> [w519]
                      n658 = Index Array(array=w518, index=w519) -> (element=w517:refnum<vi>)
                      n659 = invoke class="VI" method="Ctrl Val.Set"(reference=w517, error in=w516, "Control Name"="Connect", "Value"=FALSE) -> (error out=w515:errorcluster)  [unwired: 1 in, 4 out]
                    }
                  }
                  frame Enabled {
                  }
                }
                n660 = property on="Set Output ON All" class="Bool (strict)"("Disabled"=w508) -> ()  [unwired: 2 in, 2 out]
                n661 = property on="CurrentModulationB" class="Bool (strict)"("Disabled"=w508) -> ()  [unwired: 2 in, 2 out]
                n662 = property on="ConnectAll" class="Bool (strict)"("Disabled"=w508) -> ()  [unwired: 2 in, 2 out]
                n663 = property on="ReadFromFile" class="Bool (strict)"("Disabled"=w508) -> ()  [unwired: 2 in, 2 out]
                n664 = property on="ConnectChannel" class="Bool (strict)"("Disabled"=w508) -> ()  [unwired: 2 in, 2 out]
                n665 = property on="DisconnectChannel" class="Bool (strict)"("Disabled"=w508) -> ()  [unwired: 2 in, 2 out]
                n666 = property on="WriteToFile" class="Bool (strict)"("Disabled"=w508) -> ()  [unwired: 2 in, 2 out]
                n667 = property on="AddChannel" class="Bool (strict)"("Disabled"=w508) -> ()  [unwired: 2 in, 2 out]
                n668 = property on="SetOutputOnB" class="Bool (strict)"("Disabled"=w508) -> ()  [unwired: 2 in, 2 out]
                n669 = property on="Quit" class="Bool (strict)"("Disabled"=w508) -> ()  [unwired: 2 in, 2 out]
                n670 = property on="DeleteChannel" class="Bool (strict)"("Disabled"=w508) -> ()  [unwired: 2 in, 2 out]
                n671 = property on="SetCurrentB" class="Bool (strict)"("Disabled"=w508) -> ()  [unwired: 2 in, 2 out]
                n672 = property on="SetOutputOffB" class="Bool (strict)"("Disabled"=w508) -> ()  [unwired: 2 in, 2 out]
                n673 = property on="SetCurrentAll" class="Bool (strict)"("Disabled"=w508) -> ()  [unwired: 2 in, 2 out]
                n674 = property on="SetVoltageB" class="Bool (strict)"("Disabled"=w508) -> ()  [unwired: 2 in, 2 out]
                n675 = property on="SetVoltageAll" class="Bool (strict)"("Disabled"=w508) -> ()  [unwired: 2 in, 2 out]
                n676 = property on="DisconnectAll" class="Bool (strict)"("Disabled"=w508) -> ()  [unwired: 2 in, 2 out]
              }
              frame #1 {
                n677 = Wait (ms)(milliseconds to wait=u32 1000) -> ()  [unwired: 1 out]
              }
              frame #2 {
                n678 = local read "Measure_VI"() -> (w527:refnum<vi>[])
                n679 = Wait (ms)(milliseconds to wait=u32 250) -> ()  [unwired: 1 out]
                n680 = Array Size(array=w527) -> (size(s)=w526:i32)
                n681 = for {
                  N: w526 -> [_]
                  tunnel: w527 -> [w529]
                  i -> [w530]
                  n682 = Index Array(array=w529, index=w530) -> (element=w528:refnum<vi>)
                  n683 = invoke class="VI" method="Abort VI"(reference=w528) -> ()  [unwired: 2 in, 3 out]
                }
              }
              frame #3 {
                w532 = string[] [] ("GlobalInAdress")
                n684 = local write "NAME"(w532) -> ()
                n685 = local write "ADRESS"(w532) -> ()
                n686 = local write "Measure_VI"(refnum<vi>[] []) -> ()
              }
              frame #4 {
                n687 = Index Array(array=w533, index=0) -> (element=w537:string)
                n688 = Decimal String To Number(string=w537) -> (number=w535:i32)  [unwired: 3 out]
                n689 = for {
                  N: w535 -> [_]
                  tunnel: w533 -> [w562]
                  tunnel: [w540] -> w534 mode=indexing
                  i -> [w565]
                  n690 = Add(x=2, y=w565) -> (x+y=w564:i32)
                  n691 = Index Array(array=w562, index=w564) -> (element=w561:string)
                  n692 = Spreadsheet String To Array(format string="%s", spreadsheet string=w561, array type (2D Dbl)=string[] [] ("GlobalInAdress")) -> (array=w552:string[])  [unwired: 1 out]
                  n693 = Index Array(array=w552, index=3) -> (element=w538:string)
                  n694 = Index Array(array=w552, index=0) -> (element=w556:string)
                  n695 = Index Array(array=w552, index=1) -> (element=w557:string)
                  n696 = Index Array(array=w552, index=2) -> (element=w539:string)
                  n697 = local read "Measure_VI"() -> (w549:refnum<vi>[])
                  n698 = local read "ADRESS"() -> (w550:string[])
                  n699 = Scan From String(input string=w538, default 1=0.0 ("default value 1")) -> (output 1=w545:dbl)  [unwired: 3 in, 3 out]
                  n700 = Scan From String(input string=w539, default 1=0.0 ("default value 1")) -> (output 1=w547:dbl)  [unwired: 3 in, 3 out]
                  n701 = local read "NAME"() -> (w551:string[])
                  n702 = call "AddChannel.vi"("VIRef"=w549, "Name"=w556, "SetCurrent"=w545, "ADRESS"=w550, "NAME"=w551, "Address"=w557, "SetVoltage"=w547) -> ("NAMEOut"=w544:string[], "error out"=w541:errorcluster, "ADRESSOut"=w542:string[], "VIRefOut"=w543:refnum<vi>[])  [unwired: 1 in, 4 out]
                  n703 = local write "NAME"(w544) -> ()
                  n704 = flat-sequence {
                    tunnel: w541 -> [w567]
                    tunnel: [w567] -> w540
                    frame #0 {
                      n705 = Wait (ms)(milliseconds to wait=u32 50) -> ()  [unwired: 1 out]
                    }
                  }
                  n706 = local write "ADRESS"(w542) -> ()
                  n707 = local write "Measure_VI"(w543) -> ()
                }
              }
              frame #5 {
                w569 = u8 0 ("Disabled")
                n708 = local write "ReadFromFile"(FALSE ("ConnectChannel")) -> ()
                n709 = property on="ConnectAll" class="Bool (strict)"("Disabled"=w569) -> ()  [unwired: 2 in, 2 out]
                n710 = property on="Set Output ON All" class="Bool (strict)"("Disabled"=w569) -> ()  [unwired: 2 in, 2 out]
                n711 = property on="AddChannel" class="Bool (strict)"("Disabled"=w569) -> ()  [unwired: 2 in, 2 out]
                n712 = property on="CurrentModulationB" class="Bool (strict)"("Disabled"=w569) -> ()  [unwired: 2 in, 2 out]
                n713 = property on="DisconnectChannel" class="Bool (strict)"("Disabled"=w569) -> ()  [unwired: 2 in, 2 out]
                n714 = property on="ReadFromFile" class="Bool (strict)"("Disabled"=w569) -> ()  [unwired: 2 in, 2 out]
                n715 = property on="ConnectChannel" class="Bool (strict)"("Disabled"=w569) -> ()  [unwired: 2 in, 2 out]
                n716 = property on="DeleteChannel" class="Bool (strict)"("Disabled"=w569) -> ()  [unwired: 2 in, 2 out]
                n717 = property on="WriteToFile" class="Bool (strict)"("Disabled"=w569) -> ()  [unwired: 2 in, 2 out]
                n718 = property on="SetCurrentB" class="Bool (strict)"("Disabled"=w569) -> ()  [unwired: 2 in, 2 out]
                n719 = property on="Quit" class="Bool (strict)"("Disabled"=w569) -> ()  [unwired: 2 in, 2 out]
                n720 = property on="SetOutputOnB" class="Bool (strict)"("Disabled"=w569) -> ()  [unwired: 2 in, 2 out]
                n721 = property on="SetVoltageB" class="Bool (strict)"("Disabled"=w569) -> ()  [unwired: 2 in, 2 out]
                n722 = property on="SetOutputOffB" class="Bool (strict)"("Disabled"=w569) -> ()  [unwired: 2 in, 2 out]
                n723 = property on="SetVoltageAll" class="Bool (strict)"("Disabled"=w569) -> ()  [unwired: 2 in, 2 out]
                n724 = property on="SetCurrentAll" class="Bool (strict)"("Disabled"=w569) -> ()  [unwired: 2 in, 2 out]
                n725 = property on="DisconnectAll" class="Bool (strict)"("Disabled"=w569) -> ()  [unwired: 2 in, 2 out]
              }
            }
            n726 = Merge Errors(w506) -> (w502:errorcluster)
          }
        }
      }
      event "SetCurrentB": Value Change {
        n727 = event-data() -> ()  [unwired: 7 out]
        n728 = local write "SetCurrentB"(FALSE ("ConnectChannel")) -> ()
        n729 = property on="List of channels" class="MCListbox (strict)"() -> (error out=w573:errorcluster, "Value"=w577:i32)  [unwired: 2 in, 1 out]
        n730 = flat-sequence {
          tunnel: w577 -> [w580]
          tunnel: [w580] -> w576
          tunnel: [w578] -> w574
          tunnel: w573 -> [w578]
          tunnel: w576 -> [w582]
          tunnel: w574 -> [w581]
          tunnel: [w583] -> w572
          tunnel: [w592] -> w571
          tunnel: w572 -> [w592]
          frame #0 {
            w579 = u8 2 ("Disabled")
            n731 = property on="AddChannel" class="Bool (strict)"("Disabled"=w579) -> ()  [unwired: 2 in, 2 out]
            n732 = property on="Set Output ON All" class="Bool (strict)"("Disabled"=w579) -> ()  [unwired: 2 in, 2 out]
            n733 = property on="CurrentModulationB" class="Bool (strict)"("Disabled"=w579) -> ()  [unwired: 2 in, 2 out]
            n734 = property on="ConnectAll" class="Bool (strict)"("Disabled"=w579) -> ()  [unwired: 2 in, 2 out]
            n735 = property on="DisconnectChannel" class="Bool (strict)"("Disabled"=w579) -> ()  [unwired: 2 in, 2 out]
            n736 = property on="ReadFromFile" class="Bool (strict)"("Disabled"=w579) -> ()  [unwired: 2 in, 2 out]
            n737 = property on="Quit" class="Bool (strict)"("Disabled"=w579) -> ()  [unwired: 2 in, 2 out]
            n738 = property on="ConnectChannel" class="Bool (strict)"("Disabled"=w579) -> ()  [unwired: 2 in, 2 out]
            n739 = property on="DeleteChannel" class="Bool (strict)"("Disabled"=w579) -> ()  [unwired: 2 in, 2 out]
            n740 = property on="WriteToFile" class="Bool (strict)"("Disabled"=w579) -> ()  [unwired: 2 in, 2 out]
            n741 = property on="SetCurrentB" class="Bool (strict)"("Disabled"=w579) -> ()  [unwired: 2 in, 2 out]
            n742 = property on="SetOutputOnB" class="Bool (strict)"("Disabled"=w579) -> ()  [unwired: 2 in, 2 out]
            n743 = property on="SetVoltageB" class="Bool (strict)"("Disabled"=w579) -> ()  [unwired: 2 in, 2 out]
            n744 = property on="SetOutputOffB" class="Bool (strict)"("Disabled"=w579) -> ()  [unwired: 2 in, 2 out]
            n745 = property on="SetVoltageAll" class="Bool (strict)"("Disabled"=w579) -> ()  [unwired: 2 in, 2 out]
            n746 = property on="SetCurrentAll" class="Bool (strict)"("Disabled"=w579) -> ()  [unwired: 2 in, 2 out]
            n747 = property on="DisconnectAll" class="Bool (strict)"("Disabled"=w579) -> ()  [unwired: 2 in, 2 out]
          }
          frame #1 {
            n748 = local read "Measure_VI"() -> (w590:refnum<vi>[])
            n749 = local read "SetCurrent"() -> (w588:dbl)
            n750 = Index Array(array=w590, index=w582) -> (element=w589:refnum<vi>)
            n751 = invoke class="VI" method="Ctrl Val.Set"(reference=w589, error in=w581, "Control Name"="SetCurrent", "Value"=w588) -> (reference out=w585:refnum<vi>, error out=w584:errorcluster)  [unwired: 1 in, 3 out]
            n752 = invoke class="VI" method="Ctrl Val.Set"(reference=w585, error in=w584, "Control Name"="NeedToSetCurrent", "Value"=TRUE ("ConnectChannel")) -> (error out=w583:errorcluster)  [unwired: 1 in, 4 out]
          }
          frame #2 {
            w593 = u8 0 ("Disabled")
            n753 = property on="AddChannel" class="Bool (strict)"("Disabled"=w593) -> ()  [unwired: 2 in, 2 out]
            n754 = property on="Set Output ON All" class="Bool (strict)"("Disabled"=w593) -> ()  [unwired: 2 in, 2 out]
            n755 = property on="DisconnectChannel" class="Bool (strict)"("Disabled"=w593) -> ()  [unwired: 2 in, 2 out]
            n756 = property on="ConnectAll" class="Bool (strict)"("Disabled"=w593) -> ()  [unwired: 2 in, 2 out]
            n757 = property on="ReadFromFile" class="Bool (strict)"("Disabled"=w593) -> ()  [unwired: 2 in, 2 out]
            n758 = property on="ConnectChannel" class="Bool (strict)"("Disabled"=w593) -> ()  [unwired: 2 in, 2 out]
            n759 = property on="DeleteChannel" class="Bool (strict)"("Disabled"=w593) -> ()  [unwired: 2 in, 2 out]
            n760 = property on="Quit" class="Bool (strict)"("Disabled"=w593) -> ()  [unwired: 2 in, 2 out]
            n761 = property on="WriteToFile" class="Bool (strict)"("Disabled"=w593) -> ()  [unwired: 2 in, 2 out]
            n762 = property on="CurrentModulationB" class="Bool (strict)"("Disabled"=w593) -> ()  [unwired: 2 in, 2 out]
            n763 = property on="SetCurrentB" class="Bool (strict)"("Disabled"=w593) -> ()  [unwired: 2 in, 2 out]
            n764 = property on="SetOutputOnB" class="Bool (strict)"("Disabled"=w593) -> ()  [unwired: 2 in, 2 out]
            n765 = property on="SetVoltageB" class="Bool (strict)"("Disabled"=w593) -> ()  [unwired: 2 in, 2 out]
            n766 = property on="SetOutputOffB" class="Bool (strict)"("Disabled"=w593) -> ()  [unwired: 2 in, 2 out]
            n767 = property on="SetVoltageAll" class="Bool (strict)"("Disabled"=w593) -> ()  [unwired: 2 in, 2 out]
            n768 = property on="SetCurrentAll" class="Bool (strict)"("Disabled"=w593) -> ()  [unwired: 2 in, 2 out]
            n769 = property on="DisconnectAll" class="Bool (strict)"("Disabled"=w593) -> ()  [unwired: 2 in, 2 out]
          }
        }
      }
      event "DeleteChannel": Value Change {
        n770 = event-data() -> ()  [unwired: 7 out]
        n771 = property on="List of channels" class="MCListbox (strict)"() -> ("Value"=w597:i32)  [unwired: 2 in, 2 out]
        n772 = flat-sequence {
          tunnel: [w606] -> w598
          tunnel: w597 -> [w606]
          tunnel: [w610] -> w605
          tunnel: [w608] -> w604
          tunnel: [w609] -> w603
          tunnel: w598 -> [w608]
          tunnel: [w616] -> w602
          tunnel: w605 -> [w616]
          tunnel: [w615] -> w601
          tunnel: w604 -> [w615]
          tunnel: w603 -> [w614]
          tunnel: [w614] -> w600
          tunnel: w602 -> [w621]
          tunnel: [w620] -> w599
          tunnel: w601 -> [w620]
          tunnel: w600 -> [w619]
          tunnel: [w618] -> w595
          tunnel: w599 -> [w623]
          tunnel: [w622] -> w596
          tunnel: w595 -> [w622]
          tunnel: w596 -> [w631]
          tunnel: [w631] -> w594
          frame #0 {
            w607 = u8 2 ("Disabled")
            n773 = property on="AddChannel" class="Bool (strict)"("Disabled"=w607) -> ()  [unwired: 2 in, 2 out]
            n774 = property on="Set Output ON All" class="Bool (strict)"("Disabled"=w607) -> ()  [unwired: 2 in, 2 out]
            n775 = property on="CurrentModulationB" class="Bool (strict)"("Disabled"=w607) -> ()  [unwired: 2 in, 2 out]
            n776 = property on="ConnectAll" class="Bool (strict)"("Disabled"=w607) -> ()  [unwired: 2 in, 2 out]
            n777 = property on="DisconnectChannel" class="Bool (strict)"("Disabled"=w607) -> ()  [unwired: 2 in, 2 out]
            n778 = property on="ReadFromFile" class="Bool (strict)"("Disabled"=w607) -> ()  [unwired: 2 in, 2 out]
            n779 = property on="Quit" class="Bool (strict)"("Disabled"=w607) -> ()  [unwired: 2 in, 2 out]
            n780 = property on="ConnectChannel" class="Bool (strict)"("Disabled"=w607) -> ()  [unwired: 2 in, 2 out]
            n781 = property on="DeleteChannel" class="Bool (strict)"("Disabled"=w607) -> ()  [unwired: 2 in, 2 out]
            n782 = property on="WriteToFile" class="Bool (strict)"("Disabled"=w607) -> ()  [unwired: 2 in, 2 out]
            n783 = property on="SetCurrentB" class="Bool (strict)"("Disabled"=w607) -> ()  [unwired: 2 in, 2 out]
            n784 = property on="SetOutputOnB" class="Bool (strict)"("Disabled"=w607) -> ()  [unwired: 2 in, 2 out]
            n785 = property on="SetVoltageB" class="Bool (strict)"("Disabled"=w607) -> ()  [unwired: 2 in, 2 out]
            n786 = property on="SetOutputOffB" class="Bool (strict)"("Disabled"=w607) -> ()  [unwired: 2 in, 2 out]
            n787 = property on="SetVoltageAll" class="Bool (strict)"("Disabled"=w607) -> ()  [unwired: 2 in, 2 out]
            n788 = property on="SetCurrentAll" class="Bool (strict)"("Disabled"=w607) -> ()  [unwired: 2 in, 2 out]
            n789 = property on="DisconnectAll" class="Bool (strict)"("Disabled"=w607) -> ()  [unwired: 2 in, 2 out]
          }
          frame #1 {
            n790 = local read "Measure_VI"() -> (w612:refnum<vi>[])
            n791 = Index Array(array=w612, index=w608) -> (element=w610:refnum<vi>)
            n792 = invoke class="VI" method="Ctrl Val.Set"(reference=w610, "Control Name"="Connect", "Value"=FALSE ("OK Button")) -> (error out=w609:errorcluster)  [unwired: 2 in, 4 out]
          }
          frame #2 {
            n793 = Wait (ms)(milliseconds to wait=u32 1000) -> ()  [unwired: 1 out]
          }
          frame #3 {
            n794 = invoke class="VI" method="Abort VI"(reference=w621, error in=w619) -> (error out=w618:errorcluster)  [unwired: 1 in, 2 out]
          }
          frame #4 {
            w624 = 1 ("length")
            n795 = local read "Measure_VI"() -> (w630:refnum<vi>[])
            n796 = local read "ADRESS"() -> (w629:string[])
            n797 = local read "NAME"() -> (w625:string[])
            n798 = Delete From Array(array=w630, length=w624, index=w623) -> (array with subset deleted=w627:refnum<vi>[])  [unwired: 1 out]
            n799 = Delete From Array(array=w629, length=w624, index=w623) -> (array with subset deleted=w628:string[])  [unwired: 1 out]
            n800 = Delete From Array(array=w625, length=w624, index=w623) -> (array with subset deleted=w626:string[])  [unwired: 1 out]
            n801 = local write "ADRESS"(w628) -> ()
            n802 = local write "Measure_VI"(w627) -> ()
            n803 = local write "NAME"(w626) -> ()
          }
          frame #5 {
            w632 = u8 0 ("Disabled")
            n804 = local write "DeleteChannel"(FALSE ("DeleteChannel")) -> ()
            n805 = property on="AddChannel" class="Bool (strict)"("Disabled"=w632) -> ()  [unwired: 2 in, 2 out]
            n806 = property on="CurrentModulationB" class="Bool (strict)"("Disabled"=w632) -> ()  [unwired: 2 in, 2 out]
            n807 = property on="DisconnectChannel" class="Bool (strict)"("Disabled"=w632) -> ()  [unwired: 2 in, 2 out]
            n808 = property on="ReadFromFile" class="Bool (strict)"("Disabled"=w632) -> ()  [unwired: 2 in, 2 out]
            n809 = property on="ConnectChannel" class="Bool (strict)"("Disabled"=w632) -> ()  [unwired: 2 in, 2 out]
            n810 = property on="Quit" class="Bool (strict)"("Disabled"=w632) -> ()  [unwired: 2 in, 2 out]
            n811 = property on="DeleteChannel" class="Bool (strict)"("Disabled"=w632) -> ()  [unwired: 2 in, 2 out]
            n812 = property on="WriteToFile" class="Bool (strict)"("Disabled"=w632) -> ()  [unwired: 2 in, 2 out]
            n813 = property on="Set Output ON All" class="Bool (strict)"("Disabled"=w632) -> ()  [unwired: 2 in, 2 out]
            n814 = property on="SetCurrentB" class="Bool (strict)"("Disabled"=w632) -> ()  [unwired: 2 in, 2 out]
            n815 = property on="ConnectAll" class="Bool (strict)"("Disabled"=w632) -> ()  [unwired: 2 in, 2 out]
            n816 = property on="SetOutputOnB" class="Bool (strict)"("Disabled"=w632) -> ()  [unwired: 2 in, 2 out]
            n817 = property on="SetVoltageB" class="Bool (strict)"("Disabled"=w632) -> ()  [unwired: 2 in, 2 out]
            n818 = property on="SetOutputOffB" class="Bool (strict)"("Disabled"=w632) -> ()  [unwired: 2 in, 2 out]
            n819 = property on="SetVoltageAll" class="Bool (strict)"("Disabled"=w632) -> ()  [unwired: 2 in, 2 out]
            n820 = property on="SetCurrentAll" class="Bool (strict)"("Disabled"=w632) -> ()  [unwired: 2 in, 2 out]
            n821 = property on="DisconnectAll" class="Bool (strict)"("Disabled"=w632) -> ()  [unwired: 2 in, 2 out]
          }
        }
      }
    }
    n822 = call <vilib>:"General Error Handler.vi"("type of dialog (OK msg:1)"=u8 0 ("Disabled"), "error in (no error)"=w70) -> ()  [unwired: 14 out]
  }
  n823 = while {
    stop <- FALSE stop-if-true
    n824 = property on="AddChannel" class="Bool (strict)"() -> ("Disabled"=w641:u8)  [unwired: 2 in, 2 out]
    n825 = Wait Until Next ms Multiple(millisecond multiple=u32 50) -> ()  [unwired: 1 out]
    n826 = local read "Quit"() -> (w639:bool)
    n827 = Not(x=w639) -> (.not. x?=w638:bool)
    n828 = Equal?(x=w641, y=u8 0) -> (x = y?=w637:bool)
    n829 = And(x=w638, y=w637) -> (x .and. y?=w636:bool)
    n830 = case shown="True" w636 {
      frame False {
      }
      frame True {
        w647 = string[] [] ("GlobalInAdress")
        n831 = local read "Measure_VI"() -> (w654:refnum<vi>[])
        n832 = Array Size(array=w654) -> (size(s)=w646:i32)
        n833 = for {
          N: w646 -> [_]
          tunnel: w654 -> [w717]
          shift-right: [w659] -> w645
          shift-left: w647 -> [w656]
          shift-right: [w658] -> w644
          shift-left: w647 -> [w657]
          shift-right: [w708] -> w642
          shift-left: w647 -> [w709]
          shift-right: [w699] -> w643
          shift-left: w647 -> [w704]
          shift-right: [w702] -> w650
          shift-left: w647 -> [w684]
          shift-right: [w697] -> w649
          shift-left: w647 -> [w698]
          i -> [w680]
          w696 = "" ("Control Name")
          n834 = Index Array(array=w717, index=w680) -> (element=w683:refnum<vi>)
          n835 = invoke class="VI" method="Ctrl Val.Get"(reference=w683, "Control Name"="SetVoltageStr") -> (error out=w691:errorcluster, "Get Control Value Variant"=w707:variant)  [unwired: 2 in, 2 out]
          n836 = invoke class="VI" method="Ctrl Val.Get"(reference=w683, "Control Name"="SetCurrentStr") -> (error out=w690:errorcluster, "Get Control Value Variant"=w706:variant)  [unwired: 2 in, 2 out]
          n837 = invoke class="VI" method="Ctrl Val.Get"(reference=w683, "Control Name"="Error") -> (error out=w679:errorcluster, "Get Control Value Variant"=w685:variant)  [unwired: 2 in, 2 out]
          n838 = invoke class="VI" method="Ctrl Val.Get"(reference=w683, "Control Name"="GetCurrent") -> (error out=w693:errorcluster, "Get Control Value Variant"=w714:variant)  [unwired: 2 in, 2 out]
          n839 = invoke class="VI" method="Ctrl Val.Get"(reference=w683, "Control Name"="GetVoltage") -> (error out=w692:errorcluster, "Get Control Value Variant"=w715:variant)  [unwired: 2 in, 2 out]
          n840 = invoke class="VI" method="Ctrl Val.Get"(reference=w683, "Control Name"="Output") -> (error out=w689:errorcluster, "Get Control Value Variant"=w700:variant)  [unwired: 2 in, 2 out]
          n841 = Variant To Data(type=w696, Variant=w707) -> (data=w661:string)  [unwired: 1 in, 1 out]
          n842 = Variant To Data(type=w696, Variant=w706) -> (data=w666:string)  [unwired: 1 in, 1 out]
          n843 = Merge Errors(w679, w693, w692, w691) -> (w688:errorcluster)
          n844 = Variant To Data(type=w696, Variant=w714) -> (data=w711:string)  [unwired: 1 in, 1 out]
          n845 = Variant To Data(type=w696, Variant=w715) -> (data=w712:string)  [unwired: 1 in, 1 out]
          n846 = Variant To Data "Out"(type=w696, Variant=w700) -> (data=w686:string)  [unwired: 1 in, 1 out]
          n847 = Merge Errors(w690, w689) -> (w687:errorcluster)
          n848 = String Length(string=w661) -> (length=w662:i32)
          n849 = String Length(string=w666) -> (length=w669:i32)
          n850 = Variant To Data(type=FALSE, Variant=w685) -> (data=w655:bool)  [unwired: 1 in, 1 out]
          n851 = case shown="False" w655 {
            tunnel: w683 -> [_ w771]
            tunnel: w680 -> [w758 w764]
            tunnel: [w757 w762] -> w676
            frame False {
              n852 = Bundle(w758, "milliseconds to wait"=8) -> (w759:cluster{i32, "milliseconds to wait":i32})  [unwired: 1 in]
              n853 = property on="error" class="MCListbox (strict)"("ActiveCell"=w759, "CellBG"=u32 16777225) -> (error out=w757:errorcluster)  [unwired: 2 in, 1 out]
            }
            frame True {
              n854 = disable-structure shown="Enabled" {
                disable-tunnel: w771 -> [w787 w793]
                disable-tunnel: [w784 _] -> w767
                disable-tunnel: [w782 w793] -> w766
                disable-tunnel: [w780 _] -> w765
                disable-tunnel: w764 -> [w779 w794]
                disable-tunnel: [w778 w794] -> w763
                frame Disabled {
                  w781 = "Connect" ("Control Name")
                  n855 = invoke class="VI" method="Ctrl Val.Set"(reference=w787, "Control Name"=w781, "Value"=FALSE ("OK Button")) -> (reference out=w783:refnum<vi>, error out=w785:errorcluster)  [unwired: 2 in, 3 out]
                  n856 = flat-sequence {
                    tunnel: w785 -> [w792]
                    tunnel: [w792] -> w784
                    tunnel: w783 -> [w790]
                    tunnel: [w790] -> w782
                    tunnel: w781 -> [w789]
                    tunnel: [w789] -> w780
                    tunnel: w779 -> [w788]
                    tunnel: [w788] -> w778
                    frame #0 {
                      n857 = Wait (ms)(milliseconds to wait=u32 2000) -> ()  [unwired: 1 out]
                    }
                  }
                }
                frame Enabled {
                }
              }
              n858 = disable-structure shown="Enabled" {
                disable-tunnel: w767 -> [w775 w777]
                disable-tunnel: w766 -> [w774 _]
                disable-tunnel: w765 -> [w773 _]
                disable-tunnel: [w772 w777] -> w762
                frame Disabled {
                  n859 = invoke class="VI" method="Ctrl Val.Set"(reference=w774, error in=w775, "Control Name"=w773, "Value"=TRUE ("OK Button")) -> (error out=w772:errorcluster)  [unwired: 1 in, 4 out]
                }
                frame Enabled {
                }
              }
              n860 = Bundle(w763, "milliseconds to wait"=8) -> (w768:cluster{i32, "milliseconds to wait":i32})  [unwired: 1 in]
              n861 = property on="error" class="MCListbox (strict)"("ActiveCell"=w768, "CellBG"=u32 16711680) -> ()  [unwired: 2 in, 2 out]
            }
          }
          n862 = case shown="6, Default" w662 {
            tunnel: [4 ("milliseconds to wait") 5 ("milliseconds to wait")] -> w663
            tunnel: [0 ("milliseconds to wait") 0 ("milliseconds to wait")] -> w664
            frame 6, Default {
            }
            frame 7 {
            }
          }
          n863 = case shown="7" w669 {
            tunnel: [4 ("milliseconds to wait") 5 ("milliseconds to wait")] -> w668
            tunnel: [0 ("milliseconds to wait") 0 ("milliseconds to wait")] -> w667
            frame 6, Default {
            }
            frame 7 {
            }
          }
          n864 = Build Array (concatenate)(w656, w711) -> (w659:string[])
          n865 = Build Array (concatenate)(w657, w712) -> (w658:string[])
          n866 = Merge Errors(w688, w687, w676) -> (w682:errorcluster)
          n867 = call <vilib>:"General Error Handler.vi"("type of dialog (OK msg:1)"=u32 0 ("milliseconds to wait"), "error in (no error)"=w682) -> ()  [unwired: 9 in, 5 out]
          n868 = case shown="\"0\"" w686 {
            tunnel: ["+" ("Control Name") "" ("Control Name") "-" ("Control Name")] -> w678
            tunnel: w680 -> [w726 w731 w736]
            frame "1" {
              n869 = Bundle(w726, "milliseconds to wait"=6) -> (w728:cluster{i32, "milliseconds to wait":i32})  [unwired: 1 in]
              n870 = property on="out" class="MCListbox (strict)"("ActiveCell"=w728, "CellBG"=u32 5895331) -> ()  [unwired: 2 in, 2 out]
            }
            frame Default {
              n871 = Bundle(w731, "milliseconds to wait"=6) -> (w733:cluster{i32, "milliseconds to wait":i32})  [unwired: 1 in]
              n872 = property on="out" class="MCListbox (strict)"("ActiveCell"=w733, "CellBG"=u32 16777225) -> ()  [unwired: 2 in, 2 out]
            }
            frame "0" {
              n873 = Bundle(w736, "milliseconds to wait"=6) -> (w738:cluster{i32, "milliseconds to wait":i32})  [unwired: 1 in]
              n874 = property on="out" class="MCListbox (strict)"("ActiveCell"=w738, "CellBG"=u32 13816530) -> ()  [unwired: 2 in, 2 out]
            }
          }
          n875 = String Subset(string=w661, offset (0)=w664, length (rest)=w663) -> (substring=w660:string)
          n876 = String Subset(string=w666, offset (0)=w667, length (rest)=w668) -> (substring=w665:string)
          n877 = case shown="False" w655 {
            tunnel: ["+" ("Control Name") "-" ("Control Name")] -> w703
            tunnel: w680 -> [w742 w749]
            tunnel: w678 -> [w741 _]
            tunnel: [w741 "?" ("Control Name")] -> w677
            frame False {
              n878 = Bundle(w742, "milliseconds to wait"=7) -> (w744:cluster{i32, "milliseconds to wait":i32})  [unwired: 1 in]
              n879 = property on="active" class="MCListbox (strict)"("ActiveCell"=w744, "CellBG"=u32 5895331) -> ()  [unwired: 2 in, 2 out]
            }
            frame True {
              n880 = Bundle(w749, "milliseconds to wait"=7) -> (w755:cluster{i32, "milliseconds to wait":i32})  [unwired: 1 in]
              n881 = property on="active" class="MCListbox (strict)"("ActiveCell"=w755, "CellBG"=u32 14869218) -> (error out=w750:errorcluster)  [unwired: 2 in, 1 out]
              n882 = Bundle(w749, "milliseconds to wait"=6) -> (w748:cluster{i32, "milliseconds to wait":i32})  [unwired: 1 in]
              n883 = property on="out" class="MCListbox (strict)"(error in=w750, "ActiveCell"=w748, "CellBG"=u32 14869218) -> ()  [unwired: 1 in, 2 out]
            }
          }
          n884 = Search and Replace String(input string=w660, search string=",", replace string="." ("replace string (\"\")")) -> (result string=w673:string)  [unwired: 5 in, 3 out]
          n885 = Search and Replace String(input string=w665, search string=",", replace string="." ("replace string (\"\")")) -> (result string=w671:string)  [unwired: 5 in, 3 out]
          n886 = Build Array (concatenate)(w704, w671) -> (w699:string[])
          n887 = Build Array (concatenate)(w709, w673) -> (w708:string[])
          n888 = Build Array (concatenate)(w698, w677) -> (w697:string[])
          n889 = Build Array (concatenate)(w684, w703) -> (w702:string[])
        }
        n890 = local read "ADRESS"() -> (w652:string[])
        n891 = local read "NAME"() -> (w651:string[])
        n892 = Build Array(w651, w652, w645, w644, w643, w642, w649, w650) -> (w653:string[][])
        n893 = Transpose 2D Array(2D array=w653) -> (transposed array=w648:string[][])
        n894 = property on="List of channels" class="MCListbox (strict)"("ItemNames"=w648) -> ()  [unwired: 2 in, 2 out]
      }
    }
  }
  n895 = property on="Set Output ON All" class="Bool (strict)"("Disabled"=w38) -> (error out=w30:errorcluster)  [unwired: 2 in, 1 out]
  n896 = property on="SetCurrentAll" class="Bool (strict)"("Disabled"=w38) -> ()  [unwired: 2 in, 2 out]
  n897 = property on="AddChannel" class="Bool (strict)"("Disabled"=w38) -> (error out=w37:errorcluster)  [unwired: 2 in, 1 out]
  n898 = property on="AddChannel" class="Bool (strict)"("Disabled"=u8 0) -> ()  [unwired: 2 in, 2 out]
  n899 = local write "текущий ист."(u8 0 ("текущий ист.")) -> ()
  n900 = property on="IP" class="Str"("Value"="" ("IP")) -> ()  [unwired: 2 in, 2 out]
  n901 = property on="№" class="Str"("Value"="" ("Name")) -> ()  [unwired: 2 in, 2 out]
  n902 = local write "WriteToFile"(w41) -> ()
  n903 = local write "DisconnectChannel"(w41) -> ()
  n904 = local write "ConnectChannel"(w41) -> ()
  n905 = local write "SetCurrentB"(w41) -> ()
  n906 = local write "ReadFromFile"(w41) -> ()
  n907 = local write "AddChannel"(w41) -> ()
  n908 = local write "Quit"(w41) -> ()
  n909 = local write "SetCurrentAll"(w41) -> ()
  n910 = local write "SetVoltageAll"(w41) -> ()
  n911 = local write "DeleteChannel"(w41) -> ()
  n912 = local write "SetVoltageB"(w41) -> ()
  n913 = local write "SetOutputOnB"(w40) -> ()
  n914 = local write "ConnectAll"(w40) -> ()
  n915 = local write "SetOutputOffB"(w40) -> ()
  n916 = local write "DisconnectAll"(w40) -> ()
  n917 = local write "CurrentModulationB"(w40) -> ()
  n918 = local write "CurrentModulationOn"(w40) -> ()
  n919 = for "инициализация цветов и размера ячеек табл." {
    N: 50 -> [_]
    i -> [w797]
    n920 = flat-sequence {
      tunnel: w797 -> [w802]
      tunnel: [w802] -> w796
      tunnel: w796 -> [w841]
      tunnel: [w841] -> w795
      tunnel: w795 -> [w854]
      frame #0 {
        w798 = "Application font" ("Font Name")
        n921 = Bundle(w802, 4) -> (w814:cluster{i32, i32})  [unwired: 1 in]
        n922 = property on="active" class="MCListbox (strict)"("ActiveCell"=w814, "Height"=u32 35 ("Active Cell:Cell Size:Height"), "CellFontSize"=u16 28 ("Size")) -> ()  [unwired: 2 in, 2 out]
        n923 = Bundle(w802, 0) -> (w825:cluster{i32, i32})  [unwired: 1 in]
        n924 = Bundle(w802, 2) -> (w801:cluster{i32, i32})  [unwired: 1 in]
        n925 = Bundle(w802, 3) -> (w815:cluster{i32, i32})  [unwired: 1 in]
        n926 = Bundle(w802, 1) -> (w824:cluster{i32, i32})  [unwired: 1 in]
        n927 = Bundle(w802, 6) -> (w800:cluster{i32, i32})  [unwired: 1 in]
        n928 = Bundle(w802, 5) -> (w799:cluster{i32, i32})  [unwired: 1 in]
        n929 = property on="active" class="MCListbox (strict)"("ActiveCell"=w825, "Height"=u32 35 ("Active Cell:Cell Size:Height"), "CellFontSize"=u16 28 ("Size"), "CellFontName"=w798) -> ()  [unwired: 2 in, 2 out]
        n930 = property on="active" class="MCListbox (strict)"("ActiveCell"=w801, "Height"=u32 35 ("Active Cell:Cell Size:Height"), "CellFontSize"=u16 28 ("Size"), "CellFontName"=w798) -> ()  [unwired: 2 in, 2 out]
        n931 = property on="active" class="MCListbox (strict)"("ActiveCell"=w815, "Height"=u32 35 ("Active Cell:Cell Size:Height"), "CellFontSize"=u16 28 ("Size"), "CellFontName"=w798) -> ()  [unwired: 2 in, 2 out]
        n932 = property on="active" class="MCListbox (strict)"("ActiveCell"=w824, "Height"=u32 35 ("Active Cell:Cell Size:Height"), "CellFontSize"=u16 28 ("Size"), "CellFontName"=w798) -> ()  [unwired: 2 in, 2 out]
        n933 = property on="active" class="MCListbox (strict)"("ActiveCell"=w800, "Height"=u32 35 ("Active Cell:Cell Size:Height"), "CellFontSize"=u16 28 ("Size"), "CellFontName"=w798) -> ()  [unwired: 2 in, 2 out]
        n934 = property on="active" class="MCListbox (strict)"("ActiveCell"=w799, "Height"=u32 35 ("Active Cell:Cell Size:Height"), "CellFontSize"=u16 28 ("Size"), "CellFontName"=w798) -> ()  [unwired: 2 in, 2 out]
      }
      frame #1 {
        w837 = T4 {"Font Name"="Application font", "Size"=28, "Bold"=FALSE, "Italic"=FALSE, "Underline"=FALSE, "Strikeout"=FALSE, "Color"=6908265} ("Active Cell:Cell Font")
        w832 = T4 {"Font Name"="Application font", "Size"=30, "Bold"=TRUE, "Italic"=FALSE, "Underline"=FALSE, "Strikeout"=FALSE, "Color"=2263842} ("Active Cell:Cell Font")
        n935 = Bundle(w841, 3) -> (w828:cluster{i32, i32})  [unwired: 1 in]
        n936 = Bundle(w841, 2) -> (w831:cluster{i32, i32})  [unwired: 1 in]
        n937 = Bundle(w841, 0) -> (w839:cluster{i32, i32})  [unwired: 1 in]
        n938 = Bundle(w841, 5) -> (w835:cluster{i32, i32})  [unwired: 1 in]
        n939 = Bundle(w841, 4) -> (w834:cluster{i32, i32})  [unwired: 1 in]
        n940 = property on="active" class="MCListbox (strict)"("ActiveCell"=w828, "CellFont"=w832) -> ()  [unwired: 2 in, 2 out]
        n941 = property on="active" class="MCListbox (strict)"("ActiveCell"=w831, "CellFont"=w832) -> ()  [unwired: 2 in, 2 out]
        n942 = property on="active" class="MCListbox (strict)"("ActiveCell"=w839, "CellFont"=T4 {"Font Name"="Application font", "Size"=28, "Bold"=FALSE, "Italic"=FALSE, "Underline"=FALSE, "Strikeout"=FALSE, "Color"=0} ("Active Cell:Cell Font")) -> ()  [unwired: 2 in, 2 out]
        n943 = property on="active" class="MCListbox (strict)"("ActiveCell"=w835, "CellFont"=w837) -> ()  [unwired: 2 in, 2 out]
        n944 = property on="active" class="MCListbox (strict)"("ActiveCell"=w834, "CellFont"=w837) -> ()  [unwired: 2 in, 2 out]
      }
      frame #2 {
        w853 = T4 {"Font Name"="Application font", "Size"=28, "Bold"=FALSE, "Italic"=FALSE, "Underline"=FALSE, "Strikeout"=FALSE, "Color"=0} ("Active Cell:Cell Font")
        n945 = Bundle(w854, 6) -> (w848:cluster{i32, i32})  [unwired: 1 in]
        n946 = Bundle(w854, 8) -> (w849:cluster{i32, i32})  [unwired: 1 in]
        n947 = Bundle(w854, 7) -> (w850:cluster{i32, i32})  [unwired: 1 in]
        n948 = property on="active" class="MCListbox (strict)"("ActiveCell"=w848, "CellBG"=u32 16777225) -> (error out=w847:errorcluster)  [unwired: 2 in, 1 out]
        n949 = property on="error" class="MCListbox (strict)"("ActiveCell"=w849, "CellBG"=u32 16777225) -> ()  [unwired: 2 in, 2 out]
        n950 = property on="out" class="MCListbox (strict)"("ActiveCell"=w850, "CellBG"=u32 16777225) -> (error out=w851:errorcluster)  [unwired: 2 in, 1 out]
        n951 = property on="active" class="MCListbox (strict)"(error in=w847, "ActiveCell"=w848, "CellFont"=w853) -> ()  [unwired: 1 in, 2 out]
        n952 = property on="active" class="MCListbox (strict)"(error in=w851, "ActiveCell"=w850, "CellFont"=w853) -> ()  [unwired: 1 in, 2 out]
      }
    }
  }
  n953 = property on="SelectedBuvSetVolB" class="Bool"("DisabledEnum"=T2."Enabled" ("Disabled")) -> ()  [unwired: 2 in, 2 out]
  n954 = call <vilib>:"Application Directory.vi"() -> ("Application Directory"=w18:path)
  n955 = property on="CurrentModulationB" class="Bool (strict)"(error in=w37, "Disabled"=w38) -> (error out=w36:errorcluster)  [unwired: 1 in, 1 out]
  n956 = Build Path(base path=w18, name or relative path="BuvConfig.dat") -> (appended path=w15:path)
  n957 = property on="DisconnectAll" class="Bool (strict)"(error in=w30, "Disabled"=w38) -> (error out=w29:errorcluster)  [unwired: 1 in, 1 out]
  n958 = property on="DisconnectChannel" class="Bool (strict)"(error in=w36, "Disabled"=w38) -> (error out=w35:errorcluster)  [unwired: 1 in, 1 out]
  n959 = Open/Create/Replace File(file path (use dialog)=w15, operation (0:open)=T1."open") -> (refnum out=w13:refnum<file>, error out=w14:errorcluster)  [unwired: 4 in, 1 out]
  n960 = Read from Text File(file (use dialog)=w13, error in=w14) -> (text=w10:string, error out=w5:errorcluster)  [unwired: 2 in, 2 out]
  n961 = property on="WriteToFile" class="Bool (strict)"(error in=w29, "Disabled"=w38) -> (error out=w28:errorcluster)  [unwired: 1 in, 1 out]
  n962 = Match Pattern(string=w10, regular expression="Z" ("string")) -> (before substring=w9:string, after substring=w6:string)  [unwired: 1 in, 2 out]
  n963 = property on="SetCurrentB" class="Bool (strict)"(error in=w28, "Disabled"=w38) -> (error out=w27:errorcluster)  [unwired: 1 in, 1 out]
  n964 = property on="ConnectAll" class="Bool (strict)"(error in=w35, "Disabled"=w38) -> (error out=w34:errorcluster)  [unwired: 1 in, 1 out]
  n965 = Scan From String(input string=w6, error in=w5) -> (error out=w2:errorcluster, output 1=w7:dbl)  [unwired: 3 in, 2 out]
  n966 = local write "SelectedBuvOutVolt"(w7) -> ()
  n967 = property on="Quit" class="Bool (strict)"(error in=w27, "Disabled"=w38) -> (error out=w26:errorcluster)  [unwired: 1 in, 1 out]
  n968 = property on="ReadFromFile" class="Bool (strict)"(error in=w34, "Disabled"=w38) -> (error out=w33:errorcluster)  [unwired: 1 in, 1 out]
  n969 = property on="SetOutputOnB" class="Bool (strict)"(error in=w26, "Disabled"=w38) -> (error out=w25:errorcluster)  [unwired: 1 in, 1 out]
  n970 = property on="ConnectChannel" class="Bool (strict)"(error in=w33, "Disabled"=w38) -> (error out=w32:errorcluster)  [unwired: 1 in, 1 out]
  n971 = Scan From String(input string=w9, error in=w2, default 1=u16 0 ("default value 1")) -> (error out=w4:errorcluster, output 1=w12:u16)  [unwired: 2 in, 2 out]
  n972 = local write "SelectedBuvPhase"(w12) -> ()
  n973 = property on="SetVoltageB" class="Bool (strict)"(error in=w25, "Disabled"=w38) -> (error out=w24:errorcluster)  [unwired: 1 in, 1 out]
  n974 = property on="SetOutputOffB" class="Bool (strict)"(error in=w24, "Disabled"=w38) -> ()  [unwired: 1 in, 2 out]
  n975 = property on="DeleteChannel" class="Bool (strict)"(error in=w32, "Disabled"=w38) -> (error out=w31:errorcluster)  [unwired: 1 in, 1 out]
  n976 = case shown="No Error" w4 {
    selector: w4 -> [w855 w857]
    tunnel: [TRUE ("LoadPhase") FALSE ("LoadPhase")] -> w3
    tunnel: [w855 w857] -> w1
    frame No Error {
    }
    frame Error {
    }
  }
  "LoadPhase" <- w3
  n977 = property on="SetVoltageAll" class="Bool (strict)"(error in=w31, "Disabled"=w38) -> ()  [unwired: 1 in, 2 out]
  n978 = while {
    tunnel: w1 -> [w861]
    stop <- FALSE stop-if-true
    n979 = flat-sequence {
      tunnel: [w874] -> w869
      tunnel: [w873] -> w868
      tunnel: w861 -> [w872]
      tunnel: w869 -> [w881]
      tunnel: w868 -> [w880]
      tunnel: [w879] -> w867
      tunnel: [w878] -> w866
      tunnel: w867 -> [w940]
      tunnel: [w939] -> w865
      tunnel: w866 -> [w938]
      tunnel: [w937] -> w864
      tunnel: w865 -> [w1009]
      tunnel: w864 -> [w1008]
      tunnel: [w989] -> w863
      tunnel: [w987] -> w862
      tunnel: w863 -> [w1066]
      tunnel: w862 -> [w1063]
      frame #0 {
        n980 = TCP Open Connection(address="172.16.21.81", remote port or service name=u16 4001, timeout ms (60000)=1000, error in (no error)=w872) -> (connection ID=w873:refnum<k5>, error out=w874:errorcluster)  [unwired: 1 in]
        "Buv con ID" <- w873
      }
      frame #1 {
        n981 = case shown="No Error" w881 {
          selector: w881 -> [w883 w936]
          tunnel: w880 -> [w885 w935]
          tunnel: [w884 w936] -> w879
          tunnel: [w882 w935] -> w878
          frame No Error {
            n982 = local read "LoadVolt"() -> (w887:bool)
            n983 = Or(x="SelectedBuvSetVolB", y=w887) -> (x .or. y?=w886:bool)
            n984 = case shown="True" w886 {
              tunnel: [w890 w894] -> w882
              tunnel: [w889 w893] -> w884
              tunnel: w885 -> [w890 w901]
              tunnel: w883 -> [w889 _]
              frame False {
              }
              frame True {
                # "Пустое считывание,\nнеобх. после команды"
                # "Установка опорного напряжения"
                n985 = local read "SelectedBuvPhase"() -> (w919:u16)
                n986 = Divide(x="SelectedBuvOutVolt", y=0.125) -> (x/y=w922:dbl)
                n987 = To Unsigned Word Integer(number=w922) -> (unsigned 16bit integer=w929:u16)
                n988 = Format Into String(format string="%d", w919) -> (resulting string=w920:string, error out=w903:errorcluster)  [unwired: 2 in]
                n989 = Format Into String(format string="%.1f", "SelectedBuvOutVolt") -> (resulting string=w914:string, error out=w904:errorcluster)  [unwired: 2 in]
                n990 = Format Into String(format string="%04d", w929) -> (resulting string=w926:string, error out=w905:errorcluster)  [unwired: 2 in]
                n991 = local write "LoadVolt"(FALSE ("LoadPhase")) -> ()
                n992 = Concatenate Strings(w920, "Z" ("string"), w914) -> (w913:string)
                n993 = Merge Errors(w903, w904, w905) -> (w902:errorcluster)
                n994 = Concatenate Strings("r" ("data in"), w926) -> (w927:string)
                n995 = TCP Write(connection ID=w901, data in=w927, 9:2000 ("timeout ms (25000)")) -> (connection ID out=w924:refnum<k5>, error out=w923:errorcluster)  [unwired: 1 in, 1 out]
                n996 = call <vilib>:"Application Directory.vi"() -> ("Application Directory"=w911:path)
                n997 = flat-sequence {
                  tunnel: [w934] -> w892
                  tunnel: w924 -> [w934]
                  tunnel: [w933] -> w891
                  tunnel: w923 -> [w933]
                  frame #0 {
                    n998 = Wait (ms)(milliseconds to wait=u32 100) -> ()  [unwired: 1 out]
                  }
                }
                n999 = Build Path(base path=w911, name or relative path="BuvConfig.dat") -> (appended path=w910:path)
                n1000 = Open/Create/Replace File(file path (use dialog)=w910, error in=w902) -> (refnum out=w917:refnum<file>, error out=w916:errorcluster)  [unwired: 4 in, 1 out]
                n1001 = Write to Text File(file (use dialog)=w917, text=w913, error in=w916) -> (error out=w907:errorcluster)  [unwired: 1 in, 2 out]
                n1002 = TCP Write(connection ID=w892, data in="u", error in (no error)=w891) -> (connection ID out=w899:refnum<k5>, error out=w895:errorcluster)  [unwired: 1 in, 1 out]
                n1003 = call <vilib>:"General Error Handler.vi"("type of dialog (OK msg:1)"=u32 0 ("milliseconds to wait"), "error in (no error)"=w907) -> ()  [unwired: 9 in, 5 out]
                n1004 = TCP Read(connection ID=w899, bytes to read=11, error in (no error)=w895, 7:T5."Standard" ("mode (standard)"), 9:2000 ("timeout ms (25000)")) -> (connection ID out=w894:refnum<k5>, error out=w893:errorcluster)  [unwired: 1 out]
              }
            }
          }
          frame Error {
          }
        }
      }
      frame #2 {
        n1005 = case shown="No Error" w940 {
          selector: w940 -> [w943 w986]
          tunnel: [w944 w986] -> w939
          tunnel: w938 -> [w942 w985]
          tunnel: [w941 w985] -> w937
          frame No Error {
            n1006 = local read "LoadPhase"() -> (w946:bool)
            n1007 = Or(x="BuvPhaseSetB", y=w946) -> (x .or. y?=w945:bool)
            n1008 = case shown="True" w945 {
              tunnel: [w948 w951] -> w941
              tunnel: [w949 w950] -> w944
              tunnel: w943 -> [w949 _]
              tunnel: w942 -> [w948 w960]
              frame False {
              }
              frame True {
                # "Пустое считывание,\nнеобх. после команды"
                # "Установка фазы"
                n1009 = local write "LoadPhase"(FALSE ("LoadPhase")) -> ()
                n1010 = Format Into String(format string="%04d", "SelectedBuvPhase") -> (resulting string=w973:string)  [unwired: 2 in, 1 out]
                n1011 = Concatenate Strings("p" ("data in"), w973) -> (w979:string)
                n1012 = local read "SelectedBuvOutVolt"() -> (w972:dbl)
                n1013 = TCP Write(connection ID=w960, data in=w979, 9:2000 ("timeout ms (25000)")) -> (connection ID out=w976:refnum<k5>)  [unwired: 1 in, 2 out]
                n1014 = call <vilib>:"Application Directory.vi"() -> ("Application Directory"=w967:path)
                n1015 = Format Into String(format string="%.1f", w972) -> (resulting string=w970:string)  [unwired: 2 in, 1 out]
                n1016 = Build Path(base path=w967, name or relative path="BuvConfig.dat") -> (appended path=w966:path)
                n1017 = Open/Create/Replace File(file path (use dialog)=w966, operation (0:open)=T1."replace or create") -> (refnum out=w975:refnum<file>, error out=w974:errorcluster)  [unwired: 4 in, 1 out]
                n1018 = Concatenate Strings(w973, "Z" ("string"), w970) -> (w969:string)
                n1019 = Write to Text File(file (use dialog)=w975, text=w969, error in=w974) -> (error out=w963:errorcluster)  [unwired: 1 in, 2 out]
                n1020 = flat-sequence {
                  tunnel: [w984] -> w953
                  tunnel: w976 -> [w984]
                  tunnel: [w983] -> w952
                  tunnel: w963 -> [w983]
                  frame #0 {
                    n1021 = Wait (ms)(milliseconds to wait=u32 100) -> ()  [unwired: 1 out]
                    "LoadVolt" <- TRUE ("LoadVolt")
                  }
                }
                n1022 = TCP Write(connection ID=w953, data in="u", error in (no error)=w952) -> (connection ID out=w955:refnum<k5>, error out=w959:errorcluster)  [unwired: 1 in, 1 out]
                n1023 = TCP Read(connection ID=w955, bytes to read=11, error in (no error)=w959, 7:T5."Standard" ("mode (standard)"), 9:2000 ("timeout ms (25000)")) -> (connection ID out=w951:refnum<k5>, error out=w950:errorcluster)  [unwired: 1 out]
              }
            }
          }
          frame Error {
          }
        }
      }
      frame #3 {
        w988 = string[] [] ("GlobalInAdress")
        n1024 = case shown="No Error" w1009 {
          selector: w1009 -> [w1030 w1061]
          tunnel: w1008 -> [w1036 w1060]
          tunnel: [w1034 "*"] -> w996
          tunnel: [w1033 w1061] -> w990
          tunnel: [w1032 w1060] -> w989
          frame No Error {
            n1025 = TCP Write(connection ID=w1036, data in="u", error in (no error)=w1030) -> (connection ID out=w1038:refnum<k5>, error out=w1042:errorcluster)  [unwired: 1 in, 1 out]
            n1026 = TCP Read(connection ID=w1038, bytes to read=11, error in (no error)=w1042, 7:T5."CRLF" ("mode (standard)"), 9:2000 ("timeout ms (25000)")) -> (connection ID out=w1031:refnum<k5>, data out=w1035:string, error out=w1043:errorcluster)
            n1027 = case shown="No Error" w1043 {
              selector: w1043 -> [_ w1058]
              tunnel: [w1053 "-"] -> w1034
              tunnel: w1035 -> [w1046 _]
              tunnel: [w1045 w1058] -> w1033
              tunnel: [w1044 w1057] -> w1032
              tunnel: w1031 -> [w1044 w1057]
              frame No Error {
                n1028 = Match Pattern(string=w1046, regular expression="=") -> (after substring=w1047:string)  [unwired: 1 in, 3 out]
                n1029 = Scan From String(format string="%f", input string=w1047, default 1=0.0 ("default value 1")) -> (error out=w1049:errorcluster, output 1=w1052:dbl)  [unwired: 2 in, 2 out]
                n1030 = Multiply(x=w1052, y=0.125) -> (x*y=w1051:dbl)
                n1031 = Format Into String(format string="%.1f", error in=w1049, w1051) -> (resulting string=w1053:string, error out=w1045:errorcluster)  [unwired: 1 in]
              }
              frame Error {
              }
            }
          }
          frame Error {
          }
        }
        n1032 = case shown="No Error" w990 {
          selector: w990 -> [w1014 w1024]
          tunnel: ["-" ("Control Name") "+" ("Control Name")] -> w993
          tunnel: [w1014 w1024] -> w987
          frame Error {
            n1033 = Bundle("milliseconds to wait"=0, "milliseconds to wait"=4) -> (w1012:T6)  [unwired: 1 in]
            n1034 = property on="Buv Table" class="MCListbox (strict)"("ActiveCell"=w1012, "CellBG"=u32 16725248) -> ()  [unwired: 2 in, 2 out]
            n1035 = Bundle("milliseconds to wait"=0, "milliseconds to wait"=3) -> (w1016:T6)  [unwired: 1 in]
            n1036 = property on="Buv Table" class="MCListbox (strict)"("ActiveCell"=w1016, "CellBG"=u32 13816530) -> ()  [unwired: 2 in, 2 out]
          }
          frame No Error {
            n1037 = Bundle("milliseconds to wait"=0, "milliseconds to wait"=4) -> (w1023:T6)  [unwired: 1 in]
            n1038 = property on="Buv Table" class="MCListbox (strict)"("ActiveCell"=w1023, "CellBG"=u32 16448250) -> ()  [unwired: 2 in, 2 out]
            n1039 = Bundle("milliseconds to wait"=0, "milliseconds to wait"=3) -> (w1025:T6)  [unwired: 1 in]
            n1040 = property on="Buv Table" class="MCListbox (strict)"("ActiveCell"=w1025, "CellBG"=u32 5895331) -> ()  [unwired: 2 in, 2 out]
          }
        }
        n1041 = property on="SelectedBuvOutVolt" class="DigNum (strict)"() -> ("Value"=w1003:dbl)  [unwired: 2 in, 2 out]
        n1042 = Format Into String(format string="%.1f", w1003) -> (resulting string=w1001:string)  [unwired: 2 in, 1 out]
        n1043 = Build Array (concatenate)(w993, string[] [] ("GlobalInAdress")) -> (w991:string[])
        n1044 = Build Array (concatenate)(w1001, string[] [] ("GlobalInAdress")) -> (w1000:string[])
        n1045 = Build Array (concatenate)(w996, string[] [] ("GlobalInAdress")) -> (w995:string[])
        n1046 = Build Array (concatenate)("1" ("address"), string[] [] ("GlobalInAdress")) -> (w1006:string[])
        n1047 = Build Array(w988, w988) -> (w998:string[][])
        n1048 = Build Array (concatenate)(w1006, w995, w1000, w991, w998) -> (w1004:string[][])
        n1049 = Transpose 2D Array(2D array=w1004) -> (transposed array=w1005:string[][])
        n1050 = property on="Buv Table" class="MCListbox (strict)"("ItemNames"=w1005) -> ()  [unwired: 2 in, 2 out]
      }
      frame #4 {
        n1051 = case shown="Error" w1063 {
          frame No Error {
          }
          frame Error {
            w1067 = TRUE ("LoadPhase")
            n1052 = local write "LoadPhase"(w1067) -> ()
            n1053 = local write "LoadVolt"(w1067) -> ()
          }
        }
        n1054 = TCP Close Connection(connection ID=w1066) -> (error out=w1065:errorcluster)  [unwired: 2 in, 1 out]
        n1055 = call <vilib>:"General Error Handler.vi"("type of dialog (OK msg:1)"=0 ("milliseconds to wait"), "error in (no error)"=w1065) -> ()  [unwired: 9 in, 5 out]
      }
    }
    n1056 = Wait Until Next ms Multiple(millisecond multiple=u32 70) -> ()  [unwired: 1 out]
    n1057 = Not(x="SetPhaseEn") -> (.not. x?=w859:bool)
    n1058 = property on="BuvPhaseSetB" class="Bool"("Visible"=w859) -> ()  [unwired: 2 in, 2 out]
    n1059 = property on="SelectedBuvPhase" class="DigNum (strict)"("Visible"=w859) -> ()  [unwired: 2 in, 2 out]
  }
  "Measure_VI" <- refnum<vi>[] []
  "ADRESS" <- string[] [] ("GlobalInAdress")
  "NAME" <- string[] [] ("GlobalInAdress")
  "CURRENTSET" <- dbl[] [] ("GlobalInAdress")
